vi "TestHarnessDPL-SCPI.vi"() -> ()   [LabVIEW 2025]
uses:
  Program Files/National Instruments/LabVIEW 2024/vi.lib/SmarAct/SmarActCTL/SA_CTL.lvclass
  <vilib>/Utility/miscctls.llb/LVMajorAndMinorColorsTypeDef.ctl
  <vilib>/Analysis/1siggen.llb/Ramp Pattern by Samples.vi
  <vilib>/Analysis/1siggen.llb/Ramp Pattern by Delta.vi
  <vilib>/Analysis/NI_AALBase.lvlib
  <userlib>/_OpenG.lib/time/time.llb/openg_time.lvlib
  instr.lib/Detector SCPI/Detector SCPI.lvlib
  <vilib>/Analysis/NI_AALPro.lvlib
  <vilib>/platform/TimedLoop/XDataNode/XDataNode.xnode
  <vilib>/Platform/TimedLoop/XDataNode/nitl_modes.ctl
  <vilib>/Platform/TimedLoop/XDataNode/XDNodeRunTimeDep.lvlib
  <vilib>/Platform/TimedLoop/XDataNode/wakeup.ctl
  <vilib>/Platform/TimedLoop/XDataNode/timing_clust.ctl
  instr.lib/Keithley 24XX/Keithley 24XX.lvlib
panel:
  out "Ref":dbl[](array[numeric])
  out "SweepData":dbl[][](array[numeric])
  in  "Exit":bool
  out "PositionerStatus":T1={"Moving"=FALSE, "CL Active"=FALSE, "Calibrating"=FALSE, "Referencing"=FALSE, "Delayed Move"=FALSE, "Sensor Present"=TRUE, "Is Calibrated"=TRUE, "Is Referenced"=TRUE, "End Stop"=FALSE, "Ranger Limit"=FALSE, "Following Limit"=FALSE, "Movement Fail"=FALSE, "Is Streaming"=FALSE, "Overload"=FALSE, "Over Temp"=FALSE, "Reference Mark"=FALSE, "Is Phased"=FALSE, "Positioner Fault"=FALSE, "Amplifier Enabled"=TRUE, "In Position"=FALSE, "Brake Enabled"=FALSE}
  out "ChannelState":i32=262368 format="%x"
  in  "Measurement Mode":T2(tab)=enum."Stage Calibration"
  in  "Device Locator":string(combo)="network:sn:MCS2-00005242"
  in  "findDevices":bool caption="Find Devices"
  in  "connect":bool
  out "connected":bool=TRUE
  out "Error Out":errorcluster
  in  "calibrate":bool
  in  "reference":bool
  in  "moveValue":i64=-10400000000 caption="Move Abs (µm)"
  in  "moveMode":u16(ring) caption="Move Mode" items=["CL_ABS", "CL_REL", "SCAN_ABS", "SCAN_REL", "STEP"]
  in  "move":bool
  in  "actuatorMode":enum32{"0", "1"}(radio)
  out "MCSChannel":i8
  out "Position (µm)":dbl=-7999576013.0
  in  "MoveStage":bool
  in  "Move To (mm)":dbl min=-13.5 max=13.5
  in  "Enable":bool=TRUE
  in  "Positioner\n Delay (ms)":u16(ring)=2 items=["1", "2", "5", "10", "20", "50", "100", "200", "500"]
  in  "Delay(mS)":u32=5
  out "Elapsed (ms)":dbl=6.0
  out "Waveform Chart":dbl(graph)=-7999.576013
  out "Peak-to-Peak (µm)":dbl=0.0026870000001508743 format="%^.4g"
  out "rms (µm)":dbl=-2.7284841053187847e-12 format="%^.4g"
  in  "Recalibrate":bool
  out "Calibration":cluster{"Array":dbl[], "Array":dbl[]}(graph)
  in  "Stage\nCal":dbl[][](array[numeric])=[[1020.0, -8440.0], [1100.0, -6120.0], [1200.0, -3330.0], [1300.0, -530.0], [1400.0, 2280.0], [1500.0, 5160.0], [1600.0, 8630.0]]
  out "slope":dbl
  out "intercept":dbl
  in  "SPI Clock":i64
  in  "Oversample":i32=1000 min=1 max=4096
  in  "Power":bool=TRUE
  in  "Detector VISA":refnum<visa-resource-name>="COM4"
  out "Detector Resource":refnum<visa-resource-name>="COM4"
  out "Voltage (V)":dbl[](array[numeric])=[3.264, 0.0, 12.488, 12.77]
  out "Current (mA)":dbl[](array[numeric])=[0.0, 0.0, 21.6, -3.65]
  in  "ThrowAway":i32=100 min=1 max=10000
  out "Detector EGSE ID String":string="Aberystwyth University,Enfys Detector,#01,v0.5.0\r\n"
  in  "ResetVDACstats":bool
  out "Counts":dbl(graph)=160.194
  in  "Gain":u16(ring) items=["High", "Med", "Low"]
  in  "DAC Value":i32=2076 min=0 max=4095 step=1
  in  "Detector":u16(ring) items=["SWIR", "MWIR"]
  out "Peak-to-Peak (counts)":dbl=0.0026870000001508743 format="%^.4g"
  out "rms (counts) 2":dbl=-2.7284841053187847e-12 format="%^.4g"
  out "Mean Value (counts)":dbl
  out "Elapsed(uS)":i32
  in  "Pause":bool
  out "XY Graph":cluster{i32[], "subarray":dbl[]}(graph)
  in  "Detector 3":u16(ring) items=["SWIR", "MWIR"]
  in  "Gain 3":u16(ring) items=["High", "Med", "Low"]
  in  "Grid":bool
  in  "SetSample":bool
  in  "SetRef":bool
  in  "Dark Level":dbl
  out "End(nm)":dbl
  out "Start(nm)":dbl
  out "Sweep":cluster{"Ramp Pattern":dbl[], dbl[]}(graph)
  in  "Go":bool
  in  "Step(µm)":dbl=10.0 min=1.0 max=2000.0 step=1.0
  in  "Finish (mm)":dbl=-8.0 min=-12.0 max=12.0 step=1.0
  in  "Start (mm)":dbl=-12.0 min=-12.0 max=12.0 step=1.0
  in  "milliseconds\n to wait":u32 max=1000
  in  "Detector 2":u16(ring) items=["SWIR", "MWIR"]
  in  "Gain 2":u16(ring) items=["High", "Med", "Low"]
  out "Elapsed(s)":dbl=32.049
  out "Cursor\nlambda":dbl
  out "samples":i32
  out "Step(nm)":dbl
  out "Reference":cluster{"Ramp Pattern":dbl[], dbl[]}(graph)
  out "Reflectance":cluster{"Ramp Pattern":dbl[], dbl[]}(graph)
  in  "Abort":bool
  out "Output vs current":cluster{dbl[], dbl[]}[](graph)
  in  "ISweep":bool
  in  "NPoints":i32=10 min=10 max=10000 step=1
  in  "MaxCurrent":dbl=1e-11 min=1e-11 max=1e-06
  in  "MinCurrent":dbl=1e-12 min=1e-12 max=1e-06
  in  "CurrentSource":refnum<visa-resource-name>="B2901_SourceMeter"
  in  "Detector 4":u16(ring) items=["SWIR", "MWIR"]
  in  "SweepVDAC":bool
  in  "ISource":dbl min=-1e-06 max=1e-06
  in  "VDAC Step":i32=1 min=1 max=100
  in  "VDAC Max":i32 min=0 max=4095
  in  "VDAC Min":i32 min=0 max=4000
  in  "Detector 5":u16(ring) items=["SWIR", "MWIR"]
  out "VDAC Sweep":cluster{dbl[], dbl[]}[](graph)
  in  "Abort SweepVDAC":bool
  in  "Step":bool
  in  "Delay 1 (ms)":i32
  in  "Current 2":dbl
  in  "Current 1":dbl
  in  "Detector 6":u16(ring) items=["SWIR", "MWIR"]
  out "Step Response":cluster{dbl[], "subarray":dbl[]}(graph)
  in  "chan (0)":i32
  in  "stop":bool
  out "Handle":refnum<class "SA_CTL.lvclass">
  out "exit":bool=TRUE
  # "Stage \n(µm)"
  # "Wavelength\n (nm)"
  # "3.3V supply"
  # "Heater"
  # "+12V Supply"
  # "-12V Supply"
  # "Pause button will halt collection and display.\nThis allows graph to be printed etc."
  # "Burst mode is intended to examine behaviour of the ADC\n\nA burst of readings is recorded on the EGSE and then gathered here."
  # "Set current to Current#1. Waits for Delay 1 to stabilise, then switches to current 2 and reads 1000 readings as fast as possible"
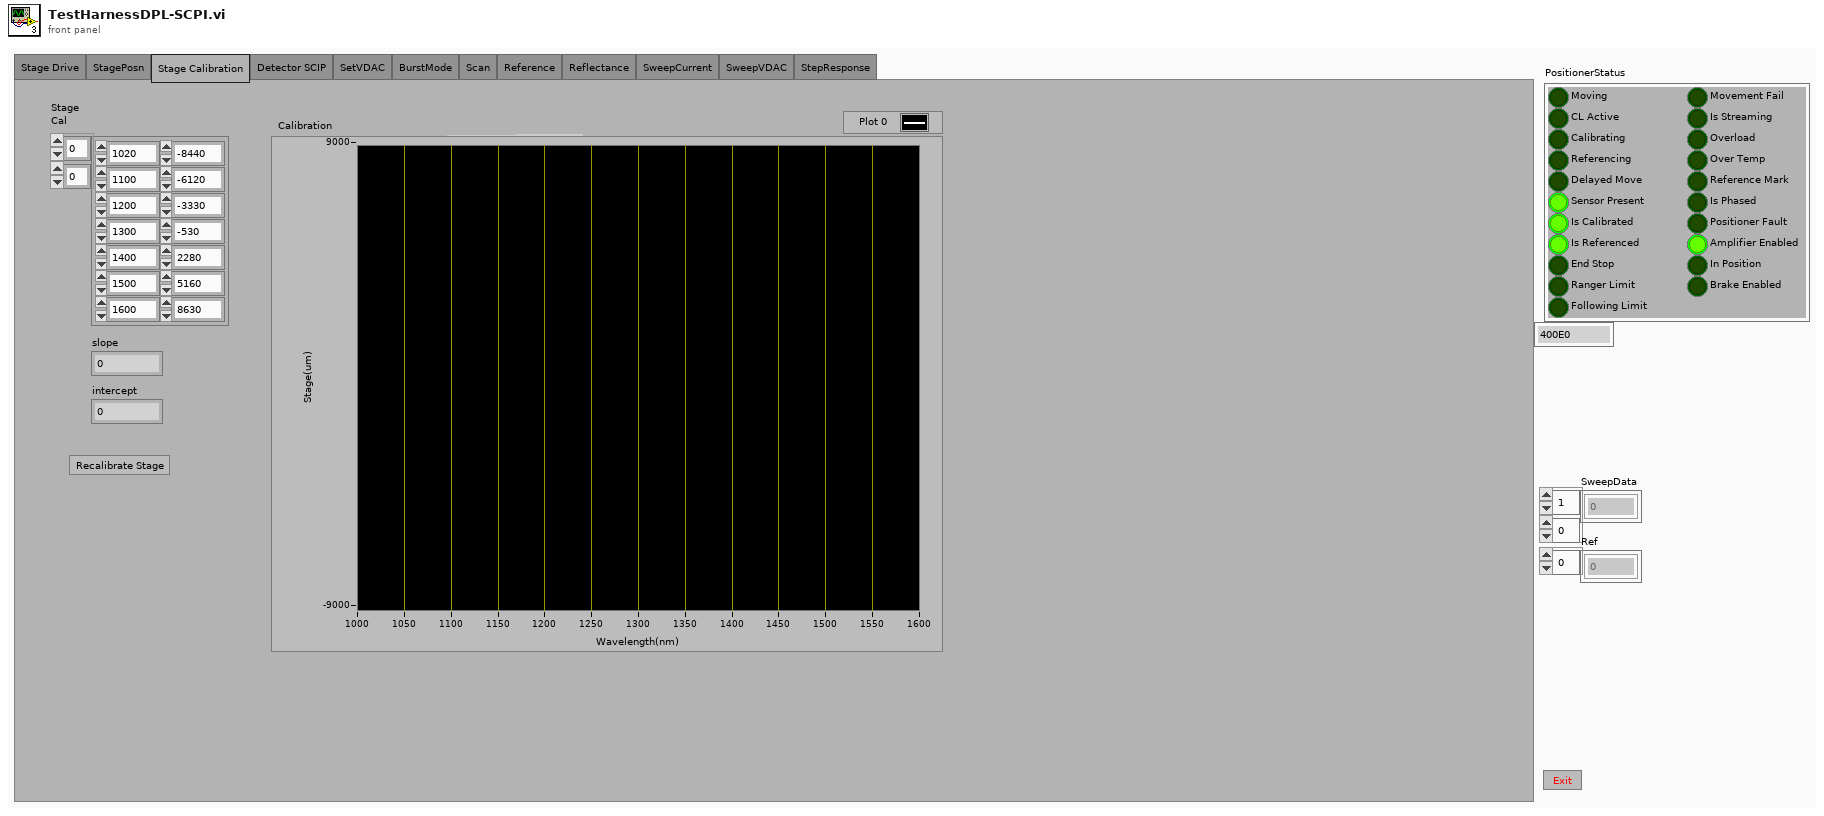
[diagram p1: front panel]
types:
  T1 = cluster{"Moving":bool, "CL Active":bool, "Calibrating":bool, "Referencing":bool, "Delayed Move":bool, "Sensor Present":bool, "Is Calibrated":bool, "Is Referenced":bool, "End Stop":bool, "Ranger Limit":bool, "Following Limit":bool, "Movement Fail":bool, "Is Streaming":bool, "Overload":bool, "Over Temp":bool, "Reference Mark":bool, "Is Phased":bool, "Positioner Fault":bool, "Amplifier Enabled":bool, "In Position":bool, "Brake Enabled":bool}
  T2 = enum32{"Stage Drive", "StagePosn", "Stage Calibration", "Detector SCIP", "SetVDAC", "BurstMode", "Scan", "Reference", "Reflectance", "SweepCurrent", "SweepVDAC", "StepResponse"}
  T3 = enum32{"Stage Drive", "StagePosn", "Stage Calibration", "Detector SCIP", "SetVDAC", "BurstMode", "Scan", "Reference", "Reflectance"}
  T4 = typedef "XDNodeRunTimeDep.lvlib/timing_clust.ctl" = cluster{"Expected End [f-1]":u64, "Actual End [f-1]":u64, "Finished Late? [f-1]":bool, "Expected End [i-1]":u64, "Actual End [i-1]":u64, "Finished Late? [i-1]":bool, "Expected Start [i]":u64, "Actual Start [i]":u64, "Expected Start [f]":u64, "Actual Start [f]":u64, "Source Name":string, "Structure Name":string, "Period":i64, "Deadline":i64, "Offset":i64, "Start":i64, "Priority":i32, "Timeout":i32, "Mode":T5, "Wakeup Reason":T6, "Error":errorcluster, "Source Type":string, "Secondary Source Type":string, "Global End Time":u64, "Global Start Time":u64, "Frame Duration":u64, "Iteration Duration":u64, "Assigned CPU":i32, "I/O Scan Engine Mode":u32}
  T5 = typedef "XDNodeRunTimeDep.lvlib/nitl_modes.ctl" = enum32{"No Change", "Process missed periods, maintain original phase", "Discard missed periods, maintain original phase", "Process missed periods, ignore original phase", "Discard missed periods, ignore original phase"}
  T6 = typedef "XDNodeRunTimeDep.lvlib/wakeup.ctl" = enum32{"Normal", "Aborted", "Asynchronous wakeup", "Timing source error", "Timed loop error", "Timeout"}
  T7 = typedef "LVMajorAndMinorColorsTypeDef.ctl" = cluster{"Major Color":u32, "Minor Color":u32}
  T8 = cluster{"Boolean array[0]":bool, "Boolean array[1]":bool, "Boolean array[2]":bool, "Boolean array[3]":bool, "Boolean array[4]":bool, "Boolean array[5]":bool, "Boolean array[6]":bool, "Boolean array[7]":bool, "Boolean array[8]":bool, "Boolean array[9]":bool, "Boolean array[10]":bool, "Boolean array[11]":bool, "Boolean array[12]":bool, "Boolean array[13]":bool, "Boolean array[14]":bool, "Boolean array[15]":bool, "Boolean array[16]":bool, "Boolean array[17]":bool, "Boolean array[18]":bool, "Boolean array[19]":bool, "Boolean array[20]":bool}
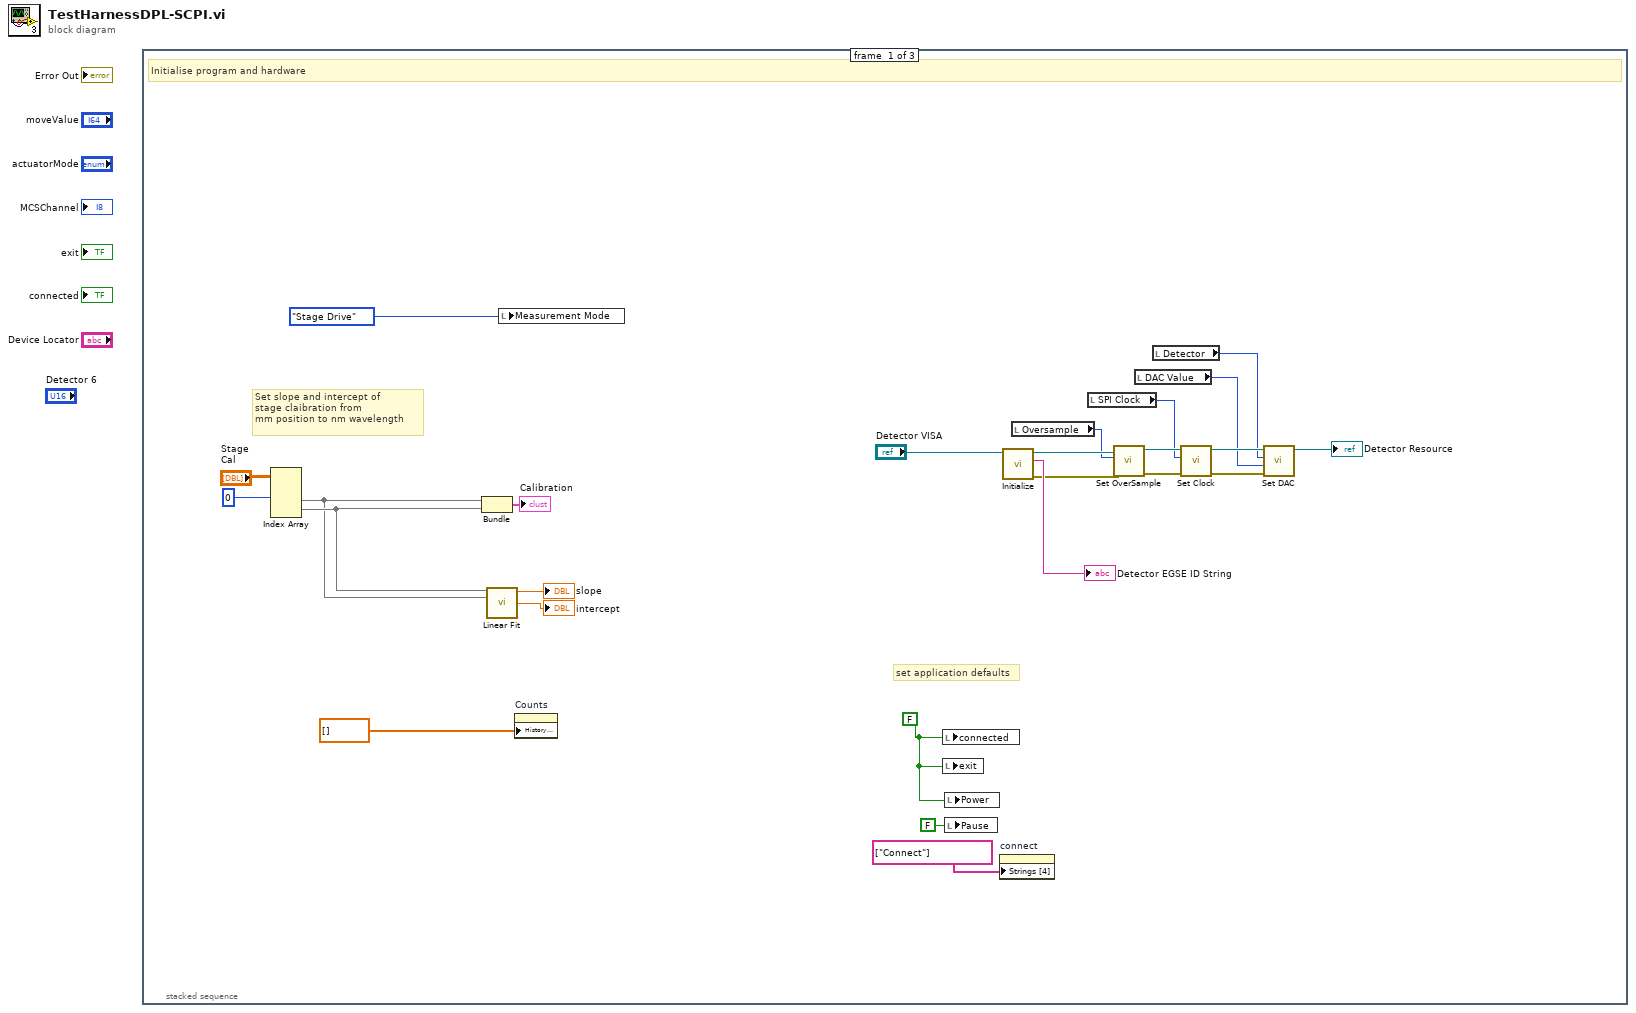
[diagram p0: block diagram]
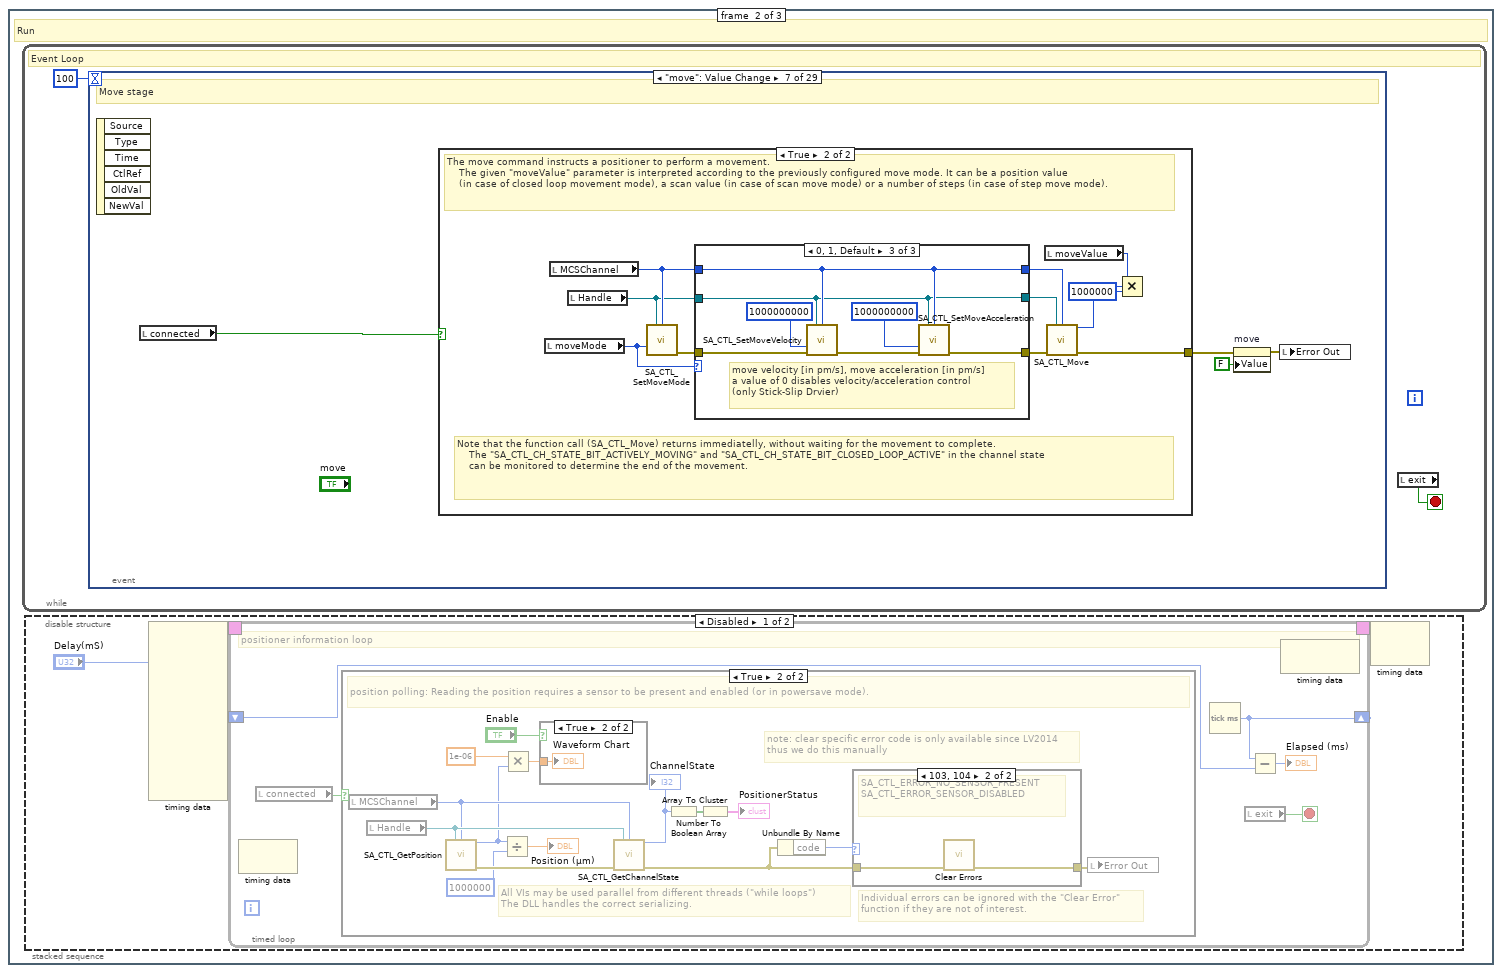
[diagram p2: hidden frame]
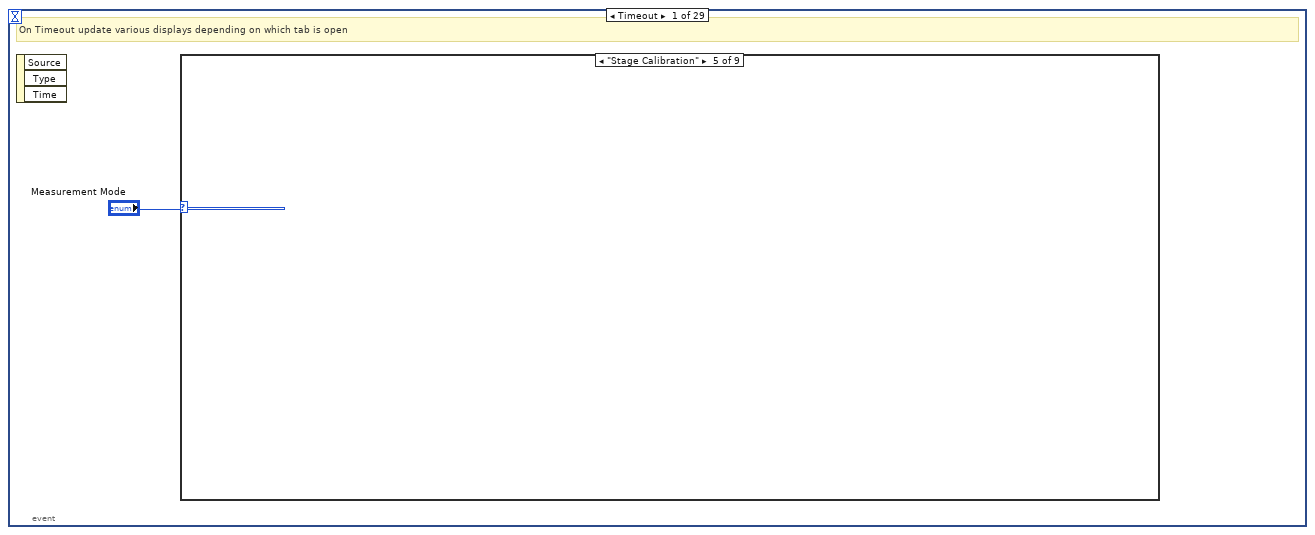
[diagram p7: hidden frame]
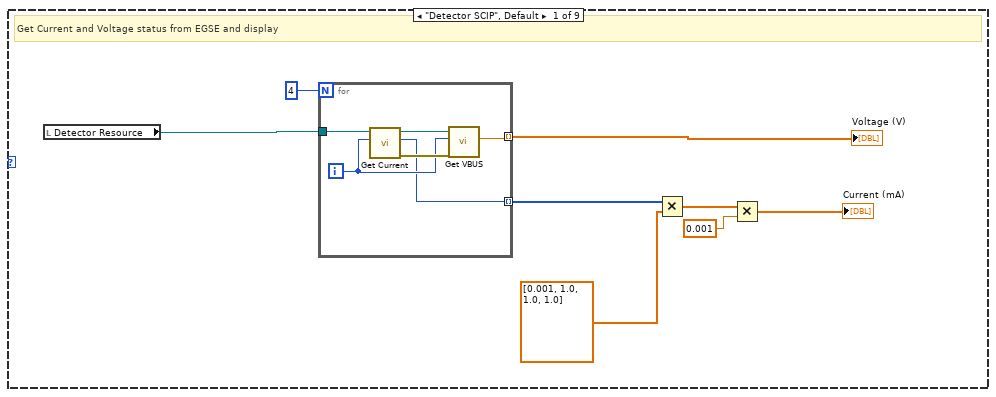
[diagram p8: hidden frame]
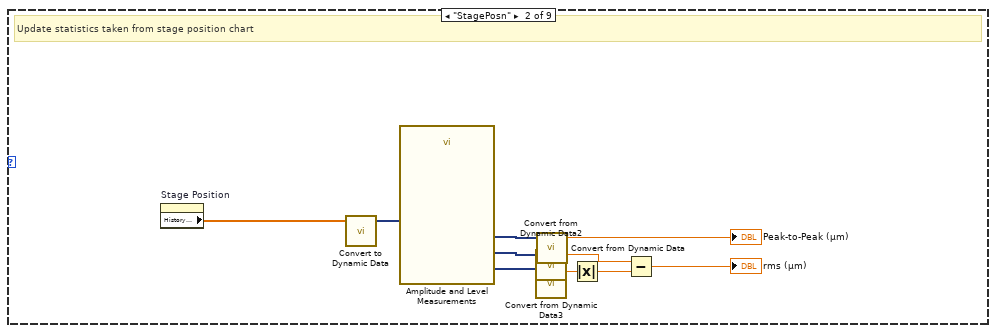
[diagram p9: hidden frame]
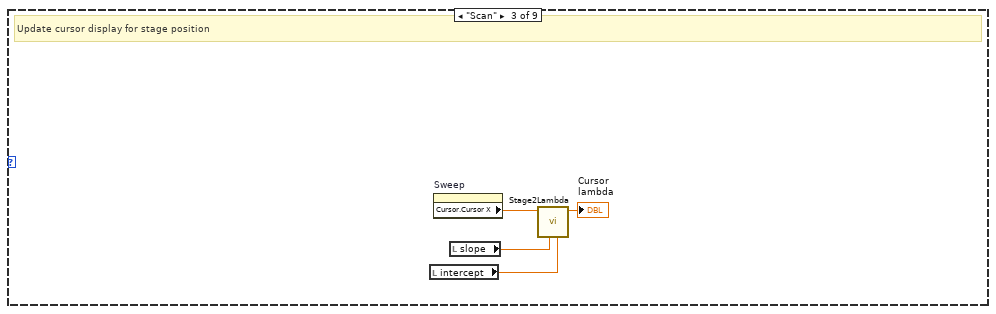
[diagram p10: hidden frame]
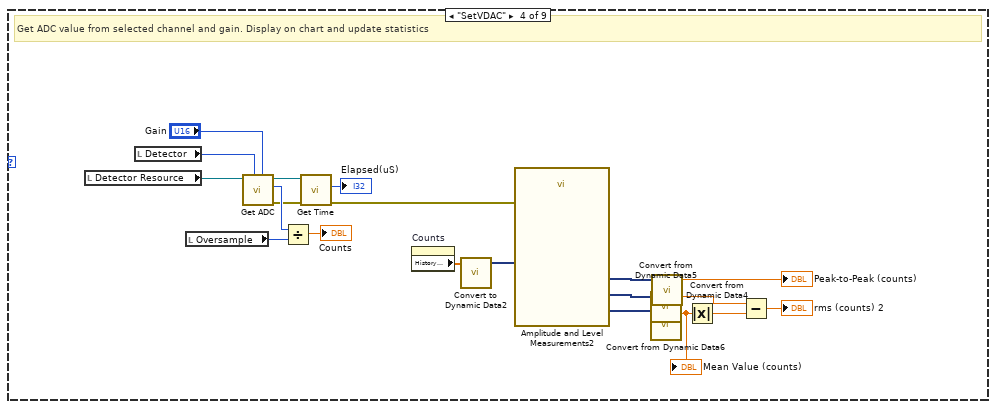
[diagram p11: hidden frame]
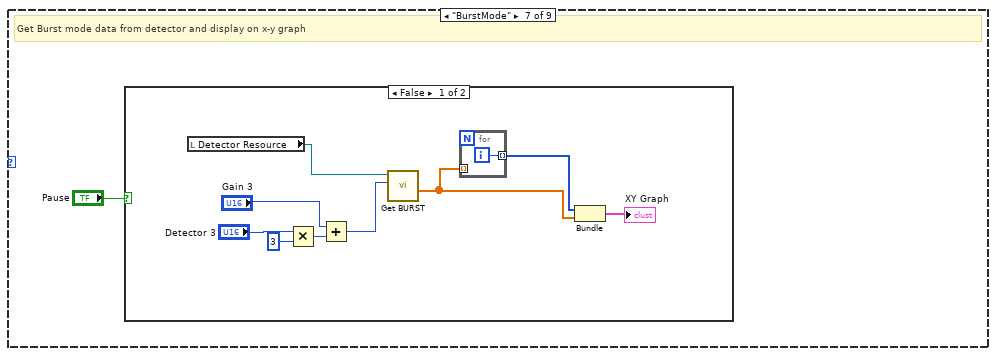
[diagram p13: hidden frame]
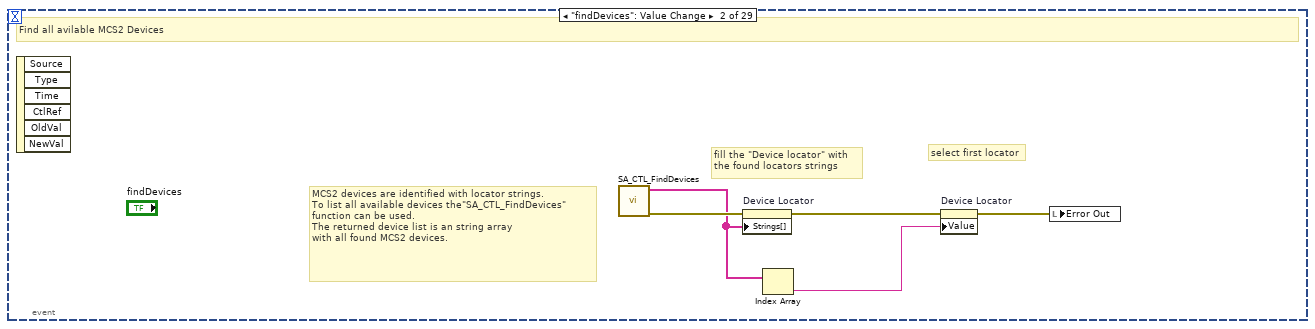
[diagram p17: hidden frame]
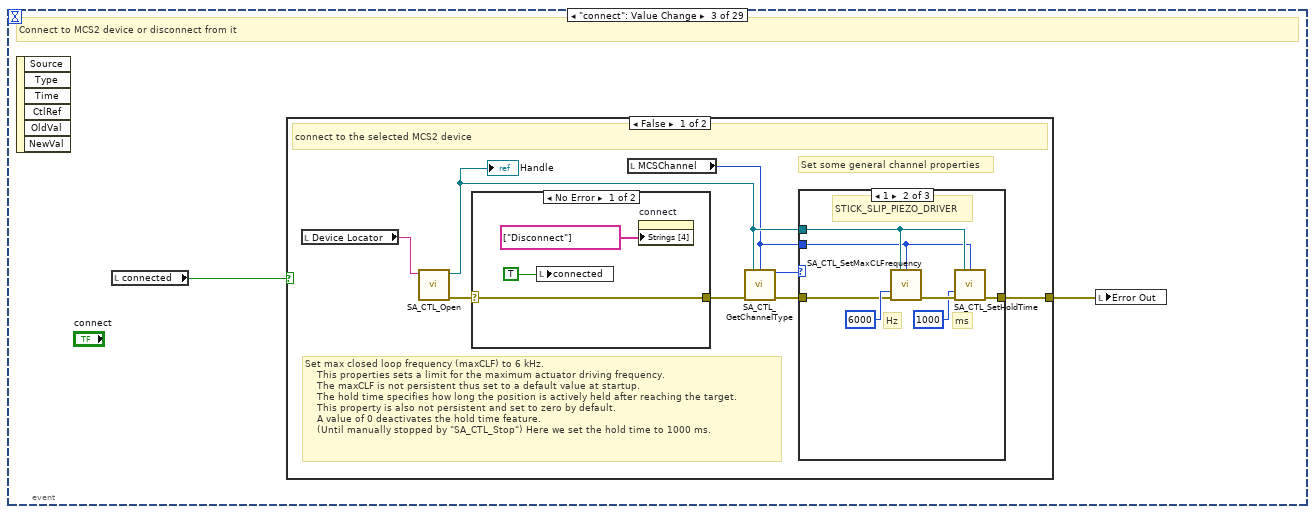
[diagram p18: hidden frame]
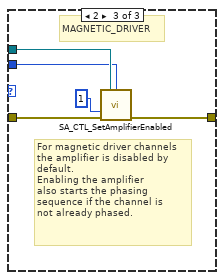
[diagram p20: hidden frame]
diagram:
  n1 = stacked-sequence {
    frame #0 {
      w21 = FALSE ("connected")
      # "Set slope and intercept of \nstage claibration from\nmm position to nm wavelength"
      # "set application defaults"
      # "Initialise program and hardware"
      n2 = Index Array(array="Stage\nCal", index (col) #1=0 ("disabled index (col)")) -> (element #1=w17:dbl[], element #2=w18:dbl[])  [unwired: 3 in]
      n3 = Bundle("Stage\nCal"=w17, "Stage\nCal"=w18) -> (→"Calibration":cluster{"Stage\nCal":dbl[], "Stage\nCal":dbl[]})  [unwired: 1 in]
      n4 = call <vilib>:"Linear Fit.vi"("Y"=w18, "X"=w17) -> ("slope"=→"slope":dbl, "intercept"=→"intercept":dbl)  [unwired: 9 in, 3 out]
      n5 = local write "Measurement Mode"(T3."Stage Drive" ("Tab Control")) -> ()
      n6 = property on="Counts" class="WFChart (strict)"("History Data"=dbl[] []) -> ()  [unwired: 2 in, 2 out]
      n7 = local write "connected"(w21) -> ()
      n8 = local write "exit"(w21) -> ()
      n9 = local write "Power"(w21) -> ()
      n10 = local write "Pause"(FALSE ("Pause")) -> ()
      n11 = property on="connect" class="Bool"("Strings [4]"=string[] ["Connect"]) -> ()  [unwired: 2 in, 2 out]
      n12 = call "Initialize.vi"("VISA resource name"="Detector VISA") -> ("error out"=w10:errorcluster, "ID String"=→"Detector EGSE ID String":string, "VISA resource name out"=w9:refnum<visa-resource-name>)  [unwired: 8 in]
      n13 = local read "Oversample"() -> (w8:i32)
      n14 = local read "SPI Clock"() -> (w3:i64)
      n15 = call "Set OverSample.vi"("error in (no error)"=w10, "oversample (0)"=w8, "VISA resource name"=w9) -> ("error out"=w7:errorcluster, "VISA resource name out"=w5:refnum<visa-resource-name>)  [unwired: 7 in]
      n16 = local read "DAC Value"() -> (w1:i32)
      n17 = local read "Detector"() -> (w2:u16)
      n18 = call "Set Clock.vi"("error in (no error)"=w7, "ClockSpeed"=w3, "VISA resource name"=w5) -> ("error out"=w6:errorcluster, "VISA resource name out"=w4:refnum<visa-resource-name>)  [unwired: 7 in]
      n19 = call "Set DAC.vi"("error in (no error)"=w6, "value (0)"=w1, "chan (0)"=w2, "VISA resource name"=w4) -> ("VISA resource name out"=→"Detector Resource":refnum<visa-resource-name>)  [unwired: 6 in, 1 out]
    }
    frame #1 {
      # "Run"
      n20 = while {
        stop <- w59 stop-if-true
        # "Event Loop"
        n21 = event shown="[6] \"move\": Value Change" {
          selector: _ -> [_ _ _ _ _ _ _ _ _ _ _ _ _ _ _ _ _ _ _ _ _ _ _ _ _ _ _ _ _]
          dyn-events: _ -> [_ _ _ _ _ _ _ _ _ _ _ _ _ _ _ _ _ _ _ _ _ _ _ _ _ _ _ _ _]
          timeout: 100 -> [_ _ _ _ _ _ _ _ _ _ _ _ _ _ _ _ _ _ _ _ _ _ _ _ _ _ _ _ _]
          event Timeout {
            # "On Timeout update various displays depending on which tab is open"
            n22 = event-data() -> ()  [unwired: 1 in, 3 out]
            n23 = case shown="\"Stage Calibration\"" "Measurement Mode" {
              frame "Detector SCIP", Default {
                # "Get Current and Voltage status from EGSE and display"
                n24 = local read "Detector Resource"() -> (w69:refnum<visa-resource-name>)
                n25 = for {
                  N: 4 -> [_]
                  tunnel: w69 -> [w75]
                  tunnel: [w71] -> w66 mode=indexing
                  tunnel: [w70] -> w67 mode=indexing
                  i -> [w72]
                  n26 = call "Get Current.vi"("chan (1)"=w72, "VISA resource name"=w75) -> ("error out"=w74:errorcluster, "output"=w71:i32, "VISA resource name out"=w73:refnum<visa-resource-name>)  [unwired: 7 in]
                  n27 = call "Get VBUS.vi"("error in (no error)"=w74, "chan (1)"=w72, "VISA resource name"=w73) -> ("output"=w70:dbl)  [unwired: 6 in, 2 out]
                }
                "Voltage (V)" <- w67
                n28 = Multiply(x=w66, y=dbl[] [0.001, 1.0, 1.0, 1.0]) -> (x*y=w63:dbl[])
                n29 = Multiply(x=w63, y=0.001) -> (x*y=→"Current (mA)":dbl[])
              }
              frame "StagePosn" {
                # "Update statistics taken from stage position chart"
                n30 = property on="Stage Position" class="WFChart (strict)"() -> ("History Data"=w85:dbl[])  [unwired: 2 in, 2 out]
                n31 = call "Convert to Dynamic Data"("Array"=w85) -> ("Dynamic Data Type"=w84:dynamicdata)  [unwired: 3 in]
                n32 = call "Amplitude and Level Measurements"("Signals"=w84) -> ("Mean (DC)"=w79:dynamicdata, "RMS"=w80:dynamicdata, "Peak to Peak"=w83:dynamicdata)  [unwired: 11 in, 1 out]
                n33 = call "Convert from Dynamic Data2"("Dynamic Data Type"=w80) -> ("Scalar"=w81:dbl)  [unwired: 3 in]
                n34 = call "Convert from Dynamic Data3"("Dynamic Data Type"=w79) -> ("Scalar"=w78:dbl)  [unwired: 3 in]
                n35 = call "Convert from Dynamic Data"("Dynamic Data Type"=w83) -> ("Scalar"=→"Peak-to-Peak (µm)":dbl)  [unwired: 3 in]
                n36 = Absolute Value(x=w78) -> (abs(x)=w76:dbl)
                n37 = Subtract(x=w81, y=w76) -> (x-y=→"rms (µm)":dbl)
              }
              frame "Scan" {
                # "Update cursor display for stage position"
                n38 = local read "intercept"() -> (w87:dbl)
                n39 = property on="Sweep" class="XYGraph (strict)"() -> ("Cursor.Cursor X"=w89:dbl)  [unwired: 2 in, 2 out]
                n40 = local read "slope"() -> (w88:dbl)
                n41 = call "Stage2Lambda.vi"("intercept"=w87, "slope"=w88, "Stage (mm)"=w89) -> ("lambda"=→"Cursor\nlambda":dbl)  [unwired: 8 in]
              }
              frame "SetVDAC" {
                # "Get ADC value from selected channel and gain. Display on chart and update statistics"
                n42 = local read "Detector Resource"() -> (w109:refnum<visa-resource-name>)
                n43 = local read "Detector"() -> (w104:u16)
                n44 = local read "Oversample"() -> (w106:i32)
                n45 = call "Get ADC.vi"("Gain"="Gain", "Detector"=w104, "VISA resource name"=w109) -> ("error out"=w102:errorcluster, "output"=w108:i32, "VISA resource name out"=w103:refnum<visa-resource-name>)  [unwired: 6 in]
                n46 = Divide(x=w108, y=w106) -> (x/y=→"Counts":dbl)
                n47 = call "Get Time.vi"("error in (no error)"=w102, "VISA resource name"=w103) -> ("error out"=w90:errorcluster, "output"=→"Elapsed(uS)":i32)  [unwired: 7 in, 1 out]
                n48 = property on="Counts" class="WFChart (strict)"() -> ("History Data"=w100:dbl[])  [unwired: 2 in, 2 out]
                n49 = call "Convert to Dynamic Data2"("Array"=w100) -> ("Dynamic Data Type"=w91:dynamicdata)  [unwired: 3 in]
                n50 = call "Amplitude and Level Measurements2"("Signals"=w91, "error in (no error)"=w90) -> ("Mean (DC)"=w96:dynamicdata, "RMS"=w95:dynamicdata, "Peak to Peak"=w92:dynamicdata)  [unwired: 10 in, 1 out]
                n51 = call "Convert from Dynamic Data5"("Dynamic Data Type"=w95) -> ("Scalar"=w94:dbl)  [unwired: 3 in]
                n52 = call "Convert from Dynamic Data6"("Dynamic Data Type"=w96) -> ("Scalar"=w97:dbl)  [unwired: 3 in]
                "Mean Value (counts)" <- w97
                n53 = call "Convert from Dynamic Data4"("Dynamic Data Type"=w92) -> ("Scalar"=→"Peak-to-Peak (counts)":dbl)  [unwired: 3 in]
                n54 = Absolute Value(x=w97) -> (abs(x)=w99:dbl)
                n55 = Subtract(x=w94, y=w99) -> (x-y=→"rms (counts) 2":dbl)
              }
              frame "Stage Calibration" {
              }
              frame "Stage Drive" {
              }
              frame "BurstMode" {
                # "Get Burst mode data from detector and display on x-y graph"
                n56 = case shown="False" "Pause" {
                  frame False {
                    n57 = local read "Detector Resource"() -> (w119:refnum<visa-resource-name>)
                    n58 = Multiply(x="Detector 3", y=u16 3) -> (x*y=w118:u16)
                    n59 = Add(x="Gain 3", y=w118) -> (x+y=w116:u16)
                    n60 = call "Get BURST.vi"("chan (0)"=w116, "VISA resource name"=w119) -> ("subarray"=w111:dbl[])  [unwired: 6 in, 3 out]
                    n61 = for {
                      tunnel: w111 -> [_] mode=indexing
                      tunnel: [w120] -> w112 mode=indexing
                      i -> [w120]
                    }
                    n62 = Bundle(w112, "subarray"=w111) -> (→"XY Graph":cluster{i32[], "subarray":dbl[]})  [unwired: 1 in]
                  }
                  frame True {
                  }
                }
              }
              frame "Reference" {
              }
              frame "Reflectance" {
              }
            }
          }
          event "findDevices": Value Change {
            # "select first locator"
            # "fill the \"Device locator\" with\nthe found locators strings"
            # "MCS2 devices are identified with locator strings.\nTo list all available devices the\"SA_CTL_FindDevices\"\nfunction can be used.\nThe returned device list is an string array \nwith all found MCS2 devices."
            # "Find all avilable MCS2 Devices"
            n63 = event-data() -> ()  [unwired: 1 in, 6 out]
            n64 = call "SA_CTL_FindDevices.vi"() -> ("error out"=w125:errorcluster, "devices"=w124:string[])  [unwired: 10 in]
            n65 = property on="Device Locator" class="CmbBox"(error in=w125, "Strings[]"=w124) -> (error out=w123:errorcluster)  [unwired: 1 in, 1 out]
            n66 = Index Array(array=w124) -> (element=w122:string)  [unwired: 1 in]
            n67 = property on="Device Locator" class="CmbBox"(error in=w123, "Value"=w122) -> (error out=w121:errorcluster)  [unwired: 1 in, 1 out]
            n68 = local write "Error Out"(w121) -> ()
          }
          event "connect": Value Change {
            # "Connect to MCS2 device or disconnect from it"
            n69 = event-data() -> ()  [unwired: 1 in, 6 out]
            n70 = local read "connected"() -> (w127:bool)
            n71 = case shown="False" w127 {
              tunnel: [w133 w153] -> w126
              frame False {
                # "Set max closed loop frequency (maxCLF) to 6 kHz.\n    This properties sets a limit for the maximum actuator driving frequency.\n    The maxCLF is not persistent thus set to a default value at startup.\n    The hold time specifies how long the position is actively held after reaching the target.\n    This property is also not persistent and set to zero by default.\n    A value of 0 deactivates the hold time feature.\n    (Until manually stopped by \"SA_CTL_Stop\") Here we set the hold time to 1000 ms."
                # "Set some general channel properties"
                # "connect to the selected MCS2 device"
                n72 = local read "Device Locator"() -> (w134:string)
                n73 = call "SA_CTL_Open.vi"("locator"=w134) -> ("error out"=w135:errorcluster, "SA_CTL_Handle"=w129:refnum<class "SA_CTL.lvclass">)  [unwired: 9 in]
                "Handle" <- w129
                n74 = case shown="No Error" w135 {
                  selector: w135 -> [w149 w152]
                  tunnel: [w149 w152] -> w132
                  frame No Error {
                    n75 = local write "connected"(TRUE ("connected")) -> ()
                    n76 = property on="connect" class="Bool"("Strings [4]"=string[] ["Disconnect"]) -> ()  [unwired: 2 in, 2 out]
                  }
                  frame Error {
                  }
                }
                n77 = local read "MCSChannel"() -> (w128:i8)
                n78 = call "SA_CTL_GetChannelType.vi"("SA_CTL_Handle"=w129, "channel"=w128, "error in (no error)"=w132) -> ("ChannelType"=w131:i32, "error out"=w130:errorcluster)  [unwired: 11 in]
                n79 = case shown="1" w131 {
                  tunnel: w129 -> [_ w140 w145]
                  tunnel: [w136 w139 w147] -> w133
                  tunnel: w128 -> [_ w138 w144]
                  tunnel: w130 -> [w136 w137 w148]
                  frame 0, Default {
                    # "unknown"
                  }
                  frame 1 {
                    # "Hz"
                    # "ms"
                    # "STICK_SLIP_PIEZO_DRIVER"
                    n80 = call "SA_CTL_SetMaxCLFrequency.vi"("SA_CTL_Handle"=w140, "channel"=w138, "MaxCLFrequency"=6000 ("MaxCLF"), "error in (no error)"=w137) -> ("error out"=w143:errorcluster)  [unwired: 11 in]
                    n81 = call "SA_CTL_SetHoldTime.vi"("SA_CTL_Handle"=w140, "channel"=w138, "HoldTime"=1000 ("MaxCLF"), "error in (no error)"=w143) -> ("error out"=w139:errorcluster)  [unwired: 11 in]
                  }
                  frame 2 {
                    # "For magnetic driver channels\nthe amplifier is disabled by\ndefault. \nEnabling the amplifier\nalso starts the phasing\nsequence if the channel is\nnot already phased."
                    # "MAGNETIC_DRIVER"
                    n82 = call "SA_CTL_SetAmplifierEnabled.vi"("SA_CTL_Handle"=w145, "channel"=w144, "AmplifierEnabled"=1, "error in (no error)"=w148) -> ("error out"=w147:errorcluster)  [unwired: 11 in]
                  }
                }
              }
              frame True {
                # "disconnect the MCS2 device"
                n83 = local read "Handle"() -> (w156:refnum<class "SA_CTL.lvclass">)
                n84 = call "SA_CTL_Close.vi"("SA_CTL_Handle"=w156) -> ("error out"=w153:errorcluster)  [unwired: 10 in]
                n85 = local write "connected"(FALSE ("connected")) -> ()
                n86 = property on="connect" class="Bool"("Strings [4]"=string[] ["Connect"]) -> ()  [unwired: 2 in, 2 out]
              }
            }
            n87 = local write "Error Out"(w126) -> ()
          }
          event "stop": Value Change {
            # "Stop - stop any movement on MCS2"
            n88 = event-data() -> ()  [unwired: 1 in, 6 out]
            n89 = local read "connected"() -> (w158:bool)
            n90 = case shown="True" w158 {
              tunnel: [_ w161] -> w157
              frame False {
              }
              frame True {
                # "Note for closed loop movements with acceleration control enabled:\n\n    The first \"stop\" command sent while moving triggers the positioner to come to a halt by decellerating to zero.\n    A second \"stop\" command triggers a hard stop (\"emergency stop\")."
                # "This command stops any ongoing movement. It also stops the hold position feature of a closed loop command."
                n91 = local read "MCSChannel"() -> (w159:i8)
                n92 = local read "Handle"() -> (w160:refnum<class "SA_CTL.lvclass">)
                n93 = call "SA_CTL_Stop.vi"("SA_CTL_Handle"=w160, "channel"=w159) -> ("error out"=w161:errorcluster)  [unwired: 13 in]
              }
            }
            n94 = local write "Error Out"(w157) -> ()
          }
          event "calibrate": Value Change {
            # "Calibratre MCS2"
            n95 = event-data() -> ()  [unwired: 1 in, 6 out]
            n96 = local read "connected"() -> (w163:bool)
            n97 = case shown="True" w163 {
              tunnel: [_ w168] -> w162
              frame False {
              }
              frame True {
                # "calibration options:\nstartDirection forward"
                # "Note that the function call (SA_CTL_Calibrate) returns immediatelly, without waiting for the movement to complete.\n    The \"SA_CTL_CH_STATE_BIT_CALIBRATING\" in the channel state can be monitored to determine the end of the calibration\n    sequence. \n \n WARNING\n    During the calibration sequence the positioner performs a movement of up to several mm, make sure to not start\n    the calibration near a mechanical endstop in order to ensure proper operation."
                # "The calibration sequence is used to increase the precision of the position calculation. This function should be called once for each\n    channel if the mechanical setup changes. (e.g. a different positioner was connected to the channel, the positioner type was set to a \n    different type) The calibration data will be saved to non-volatile memory, thus it is not necessaray to perform the calibration sequence\n    on each initialization. Note: the \"SA_CTL_CH_STATE_BIT_IS_CALIBRATED\" in the channel state can be used to determine\n    if valid calibration data is stored for the specific channel."
                n98 = local read "MCSChannel"() -> (w165:i8)
                n99 = local read "Handle"() -> (w166:refnum<class "SA_CTL.lvclass">)
                n100 = call "SA_CTL_SetCalibrationOptions.vi"("SA_CTL_Handle"=w166, "channel"=w165, "CalibrationOptions"=0 ("CalibrationMode")) -> ("error out"=w167:errorcluster)  [unwired: 12 in]
                n101 = call "SA_CTL_Calibrate.vi"("handle"=w166, "channel"=w165, "error in (no error)"=w167) -> ("error out"=w168:errorcluster)  [unwired: 12 in]
              }
            }
            n102 = local write "Error Out"(w162) -> ()
          }
          event "reference": Value Change {
            # "Find reference mark on stage"
            n103 = event-data() -> ()  [unwired: 1 in, 6 out]
            n104 = local read "connected"() -> (w170:bool)
            n105 = case shown="True" w170 {
              tunnel: [_ w179] -> w169
              frame False {
              }
              frame True {
                # "Note for Stick-Slip Driver:\nSetting the acceleration to zero \ndisables the acceleration control."
                # "The reference options specifies the behaviour of the find reference sequence. The reference flags can be ORed to build the \n    reference options. By default (options = 0) the positioner returns to the position of the reference mark.\n    Note: In contrast to previous controller systems this is not mandatory. The MCS2 controller is able to find the reference\n    position \"on-the-fly\". See the MCS2 Programmer Guide for a description of the different modes.\n    Note that the  function call (SA_CTL_Reference) returns immediatelly, without waiting for the movement to complete.\n    The \"SA_CTL_CH_STATE_BIT_REFERENCING\" in the channel state can be monitored to determine the end of the referencing\n    sequence.\n    Gere we use the \"autoZero\" option to set the position to zero after the reference position was found."
                # "Since the position sensors work on an incremental base, the referencing sequence is used to establish an absolute positioner \n    reference for the positioner after system startup.\n    Note: the \"SA_CTL_CH_STATE_BIT_IS_REFERENCED\" in the channel state can be used to to decide whether it is necessary\n    to perform the referencing sequence."
                n106 = local read "MCSChannel"() -> (w174:i8)
                n107 = local read "Handle"() -> (w175:refnum<class "SA_CTL.lvclass">)
                n108 = call "SA_CTL_SetReferencingOptions.vi"("SA_CTL_Handle"=w175, "channel"=w174, "ReferencingOptions"=0 ("CalibrationMode")) -> ("error out"=w177:errorcluster)  [unwired: 12 in]
                n109 = call "SA_CTL_SetMoveVelocity.vi"("SA_CTL_Handle"=w175, "channel"=w174, "MoveVelocity"=i64 1000000000 ("FindReferenceVelocity"), "error in (no error)"=w177) -> ("error out"=w178:errorcluster)  [unwired: 11 in]
                n110 = call "SA_CTL_SetMoveAcceleration.vi"("SA_CTL_Handle"=w175, "channel"=w174, "MoveAcceleration"=i64 10000000000 ("FindReferenceAcceleration"), "error in (no error)"=w178) -> ("error out"=w176:errorcluster)  [unwired: 11 in]
                n111 = call "SA_CTL_Reference.vi"("SA_CTL_Handle"=w175, "channel"=w174, "error in (no error)"=w176) -> ("error out"=w179:errorcluster)  [unwired: 12 in]
              }
            }
            n112 = local write "Error Out"(w169) -> ()
          }
          event "move": Value Change {
            # "Move stage"
            n113 = event-data() -> ()  [unwired: 1 in, 6 out]
            n114 = local read "connected"() -> (w183:bool)
            n115 = case shown="True" w183 {
              tunnel: [_ w194] -> w182
              frame False {
              }
              frame True {
                # "Note that the function call (SA_CTL_Move) returns immediatelly, without waiting for the movement to complete.\n    The \"SA_CTL_CH_STATE_BIT_ACTIVELY_MOVING\" and \"SA_CTL_CH_STATE_BIT_CLOSED_LOOP_ACTIVE\" in the channel state \n    can be monitored to determine the end of the movement."
                # "The move command instructs a positioner to perform a movement.\n    The given \"moveValue\" parameter is interpreted according to the previously configured move mode. It can be a position value\n    (in case of closed loop movement mode), a scan value (in case of scan move mode) or a number of steps (in case of step move mode)."
                n116 = local read "moveMode"() -> (w188:u16)
                n117 = local read "MCSChannel"() -> (w191:i8)
                n118 = local read "Handle"() -> (w186:refnum<class "SA_CTL.lvclass">)
                n119 = call "SA_CTL_SetMoveMode.vi"("SA_CTL_Handle"=w186, "channel"=w191, "MoveMode"=w188) -> ("error out"=w193:errorcluster)  [unwired: 12 in]
                n120 = case shown="0, 1, Default" w188 {
                  tunnel: w193 -> [w199 w205 w212]
                  tunnel: [w196 w202 w211] -> w192
                  tunnel: w191 -> [w198 w204 w208]
                  tunnel: [w198 w204 w208] -> w190
                  tunnel: w186 -> [w197 w203 w207]
                  tunnel: [w197 w203 w207] -> w189
                  frame 2, 3 {
                    # "scan velocity [in dac increments/s]"
                    n121 = call "SA_CTL_SetScanVelocity.vi"("SA_CTL_Handle"=w197, "channel"=w198, "ScanVelocity"=i64 65535, "error in (no error)"=w199) -> ("error out"=w196:errorcluster)  [unwired: 11 in]
                  }
                  frame 4 {
                    # "step amplitude [in dac incr.]\n0 to 65535 -> 0 to 100 V"
                    # "step frequency [in Hz]\nvalid range: 1 to 20000 Hz"
                    n122 = call "SA_CTL_SetStepFrequency.vi"("SA_CTL_Handle"=w203, "channel"=w204, "StepFrequency"=1000, "error in (no error)"=w205) -> ("error out"=w206:errorcluster)  [unwired: 11 in]
                    n123 = call "SA_CTL_SetStepAmplitude.vi"("SA_CTL_Handle"=w203, "channel"=w204, "StepAmplitude"=65535, "error in (no error)"=w206) -> ("error out"=w202:errorcluster)  [unwired: 11 in]
                  }
                  frame 0, 1, Default {
                    # "move velocity [in pm/s], move acceleration [in pm/s]\na value of 0 disables velocity/acceleration control\n(only Stick-Slip Drvier)"
                    n124 = call "SA_CTL_SetMoveVelocity.vi"("SA_CTL_Handle"=w207, "channel"=w208, "MoveVelocity"=i64 1000000000 ("FindReferenceVelocity"), "error in (no error)"=w212) -> ("error out"=w213:errorcluster)  [unwired: 11 in]
                    n125 = call "SA_CTL_SetMoveAcceleration.vi"("SA_CTL_Handle"=w207, "channel"=w208, "MoveAcceleration"=i64 1000000000 ("FindReferenceVelocity"), "error in (no error)"=w213) -> ("error out"=w211:errorcluster)  [unwired: 11 in]
                  }
                }
                n126 = local read "moveValue"() -> (w187:i64)
                n127 = Multiply(x=w187, y=i64 1000000) -> (x*y=w185:i64)
                n128 = call "SA_CTL_Move.vi"("moveValue"=w185, "SA_CTL_Handle"=w189, "channel"=w190, "error in (no error)"=w192) -> ("error out"=w194:errorcluster)  [unwired: 11 in]
              }
            }
            n129 = property on="move" class="Bool (strict)"(error in=w182, "Value"=FALSE ("move")) -> (error out=w181:errorcluster)  [unwired: 1 in, 1 out]
            n130 = local write "Error Out"(w181) -> ()
          }
          event "moveMode": Value Change {
            # "Put correct text in caption of MoveValue control"
            n131 = event-data() -> ()  [unwired: 1 in, 6 out]
            n132 = Index Array(array=string[] ["Move Abs (pm)", "Move Rel (pm)", "Move Value", "Move Value", "Move (steps)"], index="moveMode") -> (element=w215:string)
            n133 = property on="moveValue" class="DigNum (strict)"("Caption.Text"=w215) -> ()  [unwired: 2 in, 2 out]
          }
          event "actuatorMode": Value Change {
            # "Set Actuator Mode - Quiet/Normal"
            n134 = event-data() -> ("NewVal"=w217:enum32{"0", "1"})  [unwired: 1 in, 5 out]
            n135 = local read "connected"() -> (w219:bool)
            n136 = case shown="True" w219 {
              tunnel: [_ w222] -> w218
              tunnel: w217 -> [_ w220]
              frame False {
              }
              frame True {
                # "The actuator mode specifies the type of driving signal generation.\n        - normal mode (0) :    the control loop generates actuator driving signals with a maximum frequency limited to the max closed loop \n                                               frequency (maxCLF).\n        - quiet mode (1):        allows positioner movement with minimal noise emission.\n    Note that this property is not available for Magnetic Driver channels."
                n137 = local read "MCSChannel"() -> (w223:i8)
                n138 = local read "Handle"() -> (w221:refnum<class "SA_CTL.lvclass">)
                n139 = call "SA_CTL_SetActuatorMode.vi"("SA_CTL_Handle"=w221, "channel"=w223, "ActuatorMode"=w220) -> ("error out"=w222:errorcluster)  [unwired: 12 in]
              }
            }
            n140 = local write "Error Out"(w218) -> ()
          }
          event "Positioner\n Delay (ms)": Value Change {
            # "Sets delay between reading stage positioner"
            n141 = event-data() -> ()  [unwired: 1 in, 6 out]
            n142 = property on="Positioner\n Delay (ms)" class="Ring (strict)"() -> ("Strings []"=w227:string[])  [unwired: 2 in, 2 out]
            n143 = Index Array(array=w227, index="Positioner\n Delay (ms)") -> (element=w226:string)
            n144 = Decimal String To Number(string=w226) -> (number=w225:i32)  [unwired: 2 in, 1 out]
            n145 = local write "Delay(mS)"(w225) -> ()
          }
          event "Power": Value Change {
            # "Use SCPI to turn power to detector board on/off"
            n146 = event-data() -> ()  [unwired: 1 in, 6 out]
            n147 = local read "Detector Resource"() -> (w229:refnum<visa-resource-name>)
            n148 = call "Set Power.vi"("Power (0)"="Power", "VISA resource name"=w229) -> ()  [unwired: 8 in, 2 out]
          }
          event "SPI Clock": Value Change {
            n149 = event-data() -> ()  [unwired: 1 in, 6 out]
            n150 = local read "Detector Resource"() -> (w231:refnum<visa-resource-name>)
            n151 = call "Set Clock.vi"("ClockSpeed"="SPI Clock", "VISA resource name"=w231) -> ()  [unwired: 8 in, 2 out]
          }
          event "ResetVDACstats": Value Change {
            # "Reset statistics on SetVDAC page"
            n152 = event-data() -> ()  [unwired: 1 in, 6 out]
            n153 = property on="Counts" class="WFChart (strict)"("History Data"=dbl[] []) -> ()  [unwired: 2 in, 2 out]
          }
          event "Recalibrate": Value Change {
            # "Update slope and intercept for stageposn<=>lambda calculations from \"Stage Cal\" control"
            n154 = event-data() -> ()  [unwired: 1 in, 6 out]
            n155 = local read "Stage\nCal"() -> (w237:dbl[][])
            n156 = Index Array(array=w237, index (col) #1=0 ("disabled index (col)")) -> (element #1=w238:dbl[], element #2=w239:dbl[])  [unwired: 3 in]
            n157 = Bundle("Stage\nCal"=w238, "Stage\nCal"=w239) -> (w235:cluster{"Stage\nCal":dbl[], "Stage\nCal":dbl[]})  [unwired: 1 in]
            n158 = call <vilib>:"Linear Fit.vi"("Y"=w239, "X"=w238) -> ("slope"=w234:dbl, "intercept"=w233:dbl)  [unwired: 9 in, 3 out]
            n159 = local write "Calibration"(w235) -> ()
            n160 = local write "slope"(w234) -> ()
            n161 = local write "intercept"(w233) -> ()
          }
          event "MoveStage": Value Change {
            # "1E9 converts mm to pm"
            # "Move stage in mm"
            n162 = event-data() -> ()  [unwired: 1 in, 6 out]
            n163 = local read "MCSChannel"() -> (w244:i8)
            n164 = local read "Handle"() -> (w240:refnum<class "SA_CTL.lvclass">)
            n165 = Multiply(x="Move To (mm)", y=1000000000.0) -> (x*y=w242:dbl)
            n166 = To Quad Integer(1:w242) -> (0:w241:i64)
            n167 = call "SA_CTL_Move.vi"("moveValue"=w241, "SA_CTL_Handle"=w240, "channel"=w244) -> ()  [unwired: 12 in, 1 out]
          }
          event "Oversample": Value Change {
            # "Change Oversample value on EGSE"
            n168 = event-data() -> ()  [unwired: 1 in, 6 out]
            n169 = local read "Detector Resource"() -> (w247:refnum<visa-resource-name>)
            n170 = call "Set OverSample.vi"("oversample (0)"="Oversample", "VISA resource name"=w247) -> ()  [unwired: 8 in, 2 out]
          }
          event "ThrowAway": Value Change {
            # "Change Throwaway value on EGSE"
            n171 = event-data() -> ()  [unwired: 1 in, 6 out]
            n172 = local read "Detector Resource"() -> (w249:refnum<visa-resource-name>)
            n173 = call "Set ThrowAway.vi"("ThrowAway (0)"="ThrowAway", "VISA resource name"=w249) -> ()  [unwired: 8 in, 2 out]
          }
          event "DAC Value": Value Change {
            # "Change offset DAC on selected channel of detector card"
            n174 = event-data() -> ()  [unwired: 1 in, 6 out]
            n175 = local read "Detector Resource"() -> (w250:refnum<visa-resource-name>)
            n176 = call "Set DAC.vi"("value (0)"="DAC Value", "chan (0)"="Detector", "VISA resource name"=w250) -> ()  [unwired: 7 in, 2 out]
          }
          event "Go": Value Change {
            # "Initiate stage sweep"
            n177 = event-data() -> ()  [unwired: 1 in, 6 out]
            n178 = case shown="True" "Go" {
              frame False {
              }
              frame True {
                n179 = property on="Sweep" class="XYGraph (strict)"("ActXScl"=0 ("Active X Scale")) -> (error out=w258:errorcluster)  [unwired: 2 in, 1 out]
                n180 = local read "MCSChannel"() -> (w270:i8)
                n181 = local read "Handle"() -> (w269:refnum<class "SA_CTL.lvclass">)
                n182 = call <userlib>:"Tick Count (ms)__ogtk.vi"("error in (no error)"=w258) -> ("error out"=w266:errorcluster, "millisecond timer value"=w263:u32)  [unwired: 9 in]
                n183 = call "SA_CTL_SetMoveVelocity.vi"("SA_CTL_Handle"=w269, "channel"=w270, "MoveVelocity"=i64 0, "error in (no error)"=w266) -> ("error out"=w274:errorcluster)  [unwired: 11 in]
                n184 = Multiply(x=0.001, y="Step(µm)") -> (x*y=w276:dbl)
                n185 = call-poly <vilib>:"Ramp Pattern.vi"("start"="Start (mm)", "end"="Finish (mm)", "delta"=w276) -> ("samples"=→"samples":i32, "Ramp Pattern"=w267:dbl[])  [unwired: 6 in, 1 out]
                n186 = call "SA_CTL_SetMoveAcceleration.vi"("SA_CTL_Handle"=w269, "channel"=w270, "MoveAcceleration"=i64 0 ("FindReferenceVelocity"), "error in (no error)"=w274) -> ("error out"=w272:errorcluster)  [unwired: 11 in]
                n187 = for {
                  tunnel: w267 -> [w314] mode=indexing
                  tunnel: w270 -> [w310]
                  tunnel: w269 -> [w309]
                  tunnel: w272 -> [w306]
                  shift-right: [w303] -> w256
                  shift-left: dbl[] [] -> [w305]
                  tunnel: w267 -> [w296]
                  tunnel: [w297] -> w265
                  tunnel: [w296] -> w257
                  n188 = property on="Sweep" class="XYGraph (strict)"() -> (error out=w295:errorcluster, "ActXScl"=w293:i32)  [unwired: 2 in, 1 out]
                  n189 = Multiply(x=1000000000.0, y=w314) -> (x*y=w312:dbl)
                  n190 = call "SA_CTL_Move.vi"("moveValue"=w312, "SA_CTL_Handle"=w309, "channel"=w310, "error in (no error)"=w306) -> ("error out"=w311:errorcluster)  [unwired: 11 in]
                  n191 = property on="Sweep" class="XYGraph (strict)"(error in=w295, "ActXScl"=0 ("Active X Scale")) -> (error out=w294:errorcluster)  [unwired: 1 in, 1 out]
                  n192 = while {
                    tunnel: w311 -> [w322]
                    tunnel: w310 -> [w321]
                    tunnel: w309 -> [w320]
                    tunnel: [w316] -> w308
                    stop <- w318 stop-if-true
                    n193 = call "SA_CTL_GetChannelState.vi"("SA_CTL_Handle"=w320, "channel"=w321, "error in (no error)"=w322) -> ("ChannelState"=w319:i32, "error out"=w316:errorcluster)  [unwired: 11 in]
                    n194 = And(x=1, y=w319) -> (x .and. y?=w315:i32)
                    n195 = Equal To 0?(x=w315) -> (x = 0?=w318:bool)
                  }
                  n196 = property on="Sweep" class="XYGraph (strict)"(error in=w294) -> (error out=w292:errorcluster, "XScale.Maximum"=w289:dbl, "XScale.Minimum"=w287:dbl)  [unwired: 1 in, 1 out]
                  n197 = local read "intercept"() -> (w285:dbl)
                  n198 = local read "slope"() -> (w284:dbl)
                  n199 = call <userlib>:"Wait (ms)__ogtk.vi"("error in (no error)"=w308, "milliseconds to wait"="milliseconds\n to wait") -> ("error out"=w298:errorcluster)  [unwired: 8 in, 1 out]
                  n200 = property on="Sweep" class="XYGraph (strict)"(error in=w292, "ActXScl"=1 ("Active X Scale")) -> (error out=w290:errorcluster)  [unwired: 1 in, 1 out]
                  n201 = local read "Detector Resource"() -> (w299:refnum<visa-resource-name>)
                  n202 = local read "Oversample"() -> (w300:i32)
                  n203 = call "Stage2Lambda.vi"("intercept"=w285, "slope"=w284, "Stage (mm)"=w289) -> ("lambda"=w288:dbl)  [unwired: 8 in]
                  n204 = call "Stage2Lambda.vi"("intercept"=w285, "slope"=w284, "Stage (mm)"=w287) -> ("lambda"=w286:dbl)  [unwired: 8 in]
                  n205 = call "Get ADC.vi"("Gain"="Gain 2", "Detector"="Detector 2", "error in (no error)"=w298, "VISA resource name"=w299) -> ("error out"=w297:errorcluster, "output"=w302:i32)  [unwired: 5 in, 1 out]
                  n206 = property on="Sweep" class="XYGraph (strict)"(error in=w290, "XScale.Maximum"=w288, "XScale.Minimum"=w286) -> (error out=w291:errorcluster)  [unwired: 1 in, 1 out]
                  n207 = Divide(x=w302, y=w300) -> (x/y=w301:dbl)
                  n208 = Build Array (concatenate)(w305, w301) -> (w303:dbl[])
                  n209 = Bundle("Ramp Pattern"=w296, w303) -> (→"Sweep":cluster{"Ramp Pattern":dbl[], dbl[]})  [unwired: 1 in]
                  n210 = property on="Sweep" class="XYGraph (strict)"(error in=w291, "ActXScl"=w293) -> ()  [unwired: 1 in, 2 out]
                }
                n211 = call <userlib>:"Tick Count (ms)__ogtk.vi"("error in (no error)"=w265) -> ("millisecond timer value"=w264:u32)  [unwired: 9 in, 1 out]
                n212 = Build Array(w257, w256) -> (→"SweepData":dbl[][])
                n213 = Subtract(x=w264, y=w263) -> (x-y=w262:u32)
                n214 = Multiply(x=0.001, y=w262) -> (x*y=→"Elapsed(s)":dbl)
              }
            }
          }
          event "Start (mm)", "Finish (mm)": Value Change {
            n215 = event-data() -> ()  [unwired: 1 in, 6 out]
            n216 = local read "slope"() -> (w327:dbl)
            n217 = local read "Start (mm)"() -> (w328:dbl)
            n218 = local read "intercept"() -> (w326:dbl)
            n219 = call "Stage2Lambda.vi"("intercept"=w326, "slope"=w327, "Stage (mm)"=w328) -> ("lambda"=→"Start(nm)":dbl)  [unwired: 8 in]
            n220 = local read "Finish (mm)"() -> (w325:dbl)
            n221 = call "Stage2Lambda.vi"("intercept"=w326, "slope"=w327, "Stage (mm)"=w325) -> ("lambda"=→"End(nm)":dbl)  [unwired: 8 in]
          }
          event "Grid": Value Change {
            # "Turn graph grid on/off"
            n222 = event-data() -> ()  [unwired: 1 in, 6 out]
            n223 = case shown="True" "Grid" {
              tunnel: [1 0] -> w333
              tunnel: [0 1] -> w332
              frame True {
              }
              frame False {
              }
            }
            n224 = property on="Sweep" class="XYGraph (strict)"() -> (error out=w331:errorcluster, "ActXScl"=w329:i32)  [unwired: 2 in, 1 out]
            n225 = property on="Sweep" class="XYGraph (strict)"(error in=w331, "ActXScl"=w333) -> (error out=w339:errorcluster)  [unwired: 1 in, 1 out]
            n226 = property on="Sweep" class="XYGraph (strict)"(error in=w339, "XScale.GridColors"=T7 {"Major Color"=0, "Minor Color"=0} ("X Scale.Grid Colors")) -> (error out=w337:errorcluster)  [unwired: 1 in, 1 out]
            n227 = property on="Sweep" class="XYGraph (strict)"(error in=w337, "ActXScl"=w332) -> (error out=w336:errorcluster)  [unwired: 1 in, 1 out]
            n228 = property on="Sweep" class="XYGraph (strict)"(error in=w336, "XScale.GridColors"=T7 {"Major Color"=10066176, "Minor Color"=5000192} ("X Scale.Grid Colors")) -> (error out=w330:errorcluster)  [unwired: 1 in, 1 out]
            n229 = property on="Sweep" class="XYGraph (strict)"(error in=w330, "ActXScl"=w329) -> ()  [unwired: 1 in, 2 out]
          }
          event "Step(µm)": Value Change {
            n230 = event-data() -> ("NewVal"=w346:dbl)  [unwired: 1 in, 5 out]
            n231 = local read "slope"() -> (w345:dbl)
            n232 = Divide(x=w346, y=w345) -> (x/y=→"Step(nm)":dbl)
          }
          event "SetRef": Value Change {
            # "Set Reference Spectrum"
            n233 = event-data() -> ()  [unwired: 1 in, 6 out]
            n234 = case shown="True" "SetRef" {
              frame False {
              }
              frame True {
                n235 = local read "SweepData"() -> (w354:dbl[][])
                n236 = Index Array(array=w354, index (row) #1=0 ("disabled index (col)")) -> (element #1=w351:dbl[], element #2=w353:dbl[])  [unwired: 3 in]
                n237 = Subtract(x=w353, y="Dark Level") -> (x-y=w350:dbl[])
                "Ref" <- w350
                n238 = Bundle("SweepData"=w351, w350) -> (→"Reference":cluster{"SweepData":dbl[], dbl[]})  [unwired: 1 in]
              }
            }
          }
          event "SetSample": Value Change {
            # "Copy current spectrum as Sample"
            n239 = event-data() -> ()  [unwired: 1 in, 6 out]
            n240 = case shown="True" "SetSample" {
              frame False {
              }
              frame True {
                n241 = local read "SweepData"() -> (w365:dbl[][])
                n242 = local read "Dark Level"() -> (w363:dbl)
                n243 = Index Array(array=w365, index (row) #1=0 ("disabled index (col)")) -> (element #1=w360:dbl[], element #2=w364:dbl[])  [unwired: 3 in]
                n244 = local read "Ref"() -> (w361:dbl[])
                n245 = Subtract(x=w364, y=w363) -> (x-y=w362:dbl[])
                n246 = Divide(x=w362, y=w361) -> (x/y=w358:dbl[])
                n247 = for {
                  tunnel: w360 -> [w369] mode=indexing
                  tunnel: [w366] -> w359 mode=indexing
                  n248 = local read "intercept"() -> (w367:dbl)
                  n249 = local read "slope"() -> (w368:dbl)
                  n250 = call "Stage2Lambda.vi"("intercept"=w367, "slope"=w368, "Stage (mm)"=w369) -> ("lambda"=w366:dbl)  [unwired: 8 in]
                }
                n251 = Bundle(w359, w358) -> (→"Reflectance":cluster{dbl[], dbl[]})  [unwired: 1 in]
              }
            }
          }
          event "ISweep": Value Change {
            n252 = event-data() -> ()  [unwired: 1 in, 6 out]
            n253 = case shown="True" "ISweep" {
              frame False {
              }
              frame True {
                w378 = u16 1 items=["Voltage", "Current"] ("Source Mode  (0: Voltage)")
                w383 = dbl[] []
                w400 = u16 1 items=["Voltage", "Current"] ("Source Mode  (0: Voltage)")
                w404 = u16 1 items=["Volts", "Current", "Resistance"] ("Function (0: Volts)")
                w406 = u16 0 items=["Volts", "Current", "Resistance"] ("Function (0: Volts)")
                n254 = call "Initialize.vi"("ID Query (True)"=FALSE, "VISA resource name"="CurrentSource") -> ("error out"=w391:errorcluster, "VISA resource name out"=w392:refnum<visa-resource-name>)  [unwired: 8 in]
                n255 = Logarithm Base 10(1:"MaxCurrent") -> (0:w382:dbl)
                n256 = Logarithm Base 10(1:"MinCurrent") -> (0:w381:dbl)
                n257 = call "Configure Measurement.vi"("error in (no error)"=w391, "Enable Auto Range (T:Enable)"=TRUE, "Function (0: Volts)"=w406, "VISA resource name"=w392) -> ("error out"=w407:errorcluster, "VISA resource name out"=w408:refnum<visa-resource-name>)  [unwired: 6 in]
                n258 = call "Configure Measurement.vi"("Manual Range (1.0)"=1e-07, "error in (no error)"=w407, "Enable Auto Range (T:Enable)"=FALSE, "Function (0: Volts)"=w404, "VISA resource name"=w408) -> ("error out"=w402:errorcluster, "VISA resource name out"=w401:refnum<visa-resource-name>)  [unwired: 5 in]
                n259 = call-poly <vilib>:"Ramp Pattern.vi"("start"=w381, "end"=w382, "samples"="NPoints") -> ("Ramp Pattern"=w385:dbl[])  [unwired: 7 in, 1 out]
                n260 = local read "Oversample"() -> (w379:i32)
                n261 = local read "Detector Resource"() -> (w384:refnum<visa-resource-name>)
                n262 = call "Configure Output.vi"("Source Mode  (0: Voltage)"=w400, "error in (no error)"=w402, "Output Level (0)"=0.0, "VISA resource name"=w401) -> ("error out"=w398:errorcluster, "VISA resource name out"=w397:refnum<visa-resource-name>)  [unwired: 6 in]
                n263 = Power Of 10(x=w385) -> (10^x=w380:dbl[])
                n264 = call "Enable Output.vi"("error in (no error)"=w398, "Enable Output (T: Enable)"=TRUE, "VISA resource name"=w397) -> ("error out"=w394:errorcluster, "VISA resource name out"=w395:refnum<visa-resource-name>)  [unwired: 7 in]
                n265 = for {
                  tunnel: w395 -> [w444]
                  tunnel: w394 -> [w445]
                  tunnel: w380 -> [w443] mode=indexing
                  tunnel: [w441] -> w377
                  tunnel: [w432] -> w375
                  shift-right: [w436] -> _
                  shift-left: w383 -> [w438]
                  tunnel: w380 -> [w423]
                  tunnel: w384 -> [w435]
                  shift-right: [w425] -> _
                  shift-left: w383 -> [w427]
                  shift-right: [w424] -> _
                  shift-left: w383 -> [w426]
                  tunnel: w379 -> [w413]
                  tunnel: "Detector 4" -> [w411]
                  stop <- "Abort" stop-if-true
                  w428 = u16 2 items=["High", "Med", "Low"] ("Gain")
                  w429 = u16 1 items=["High", "Med", "Low"] ("Gain")
                  w439 = u16 0 items=["High", "Med", "Low"] ("Gain")
                  w442 = u16 1 items=["Voltage", "Current"] ("Source Mode  (0: Voltage)")
                  n266 = call "Configure Output.vi"("Source Mode  (0: Voltage)"=w442, "error in (no error)"=w445, "Output Level (0)"=w443, "VISA resource name"=w444) -> ("error out"=w440:errorcluster, "VISA resource name out"=w441:refnum<visa-resource-name>)  [unwired: 6 in]
                  n267 = call "Get ADC.vi"("Gain"=w439, "Detector"=w411, "error in (no error)"=w440, "VISA resource name"=w435) -> ("error out"=w434:errorcluster, "output"=w437:i32, "VISA resource name out"=w431:refnum<visa-resource-name>)  [unwired: 5 in]
                  n268 = Divide(x=w437, y=w413) -> (x/y=w417:dbl)
                  n269 = call "Get ADC.vi"("Gain"=w429, "Detector"=w411, "error in (no error)"=w434, "VISA resource name"=w431) -> ("error out"=w433:errorcluster, "output"=w416:i32, "VISA resource name out"=w430:refnum<visa-resource-name>)  [unwired: 5 in]
                  n270 = Divide(x=w416, y=w413) -> (x/y=w415:dbl)
                  n271 = call "Get ADC.vi"("Gain"=w428, "Detector"=w411, "error in (no error)"=w433, "VISA resource name"=w430) -> ("error out"=w432:errorcluster, "output"=w412:i32)  [unwired: 5 in, 1 out]
                  n272 = Divide(x=w412, y=w413) -> (x/y=w414:dbl)
                  n273 = Build Array (concatenate)(w427, w415) -> (w425:dbl[])
                  n274 = Build Array (concatenate)(w438, w417) -> (w436:dbl[])
                  n275 = Build Array (concatenate)(w426, w414) -> (w424:dbl[])
                  n276 = Bundle(w423, w436) -> (w422:cluster{dbl[], dbl[]})  [unwired: 1 in]
                  n277 = Bundle(w423, w425) -> (w421:cluster{dbl[], dbl[]})  [unwired: 1 in]
                  n278 = Bundle(w423, w424) -> (w420:cluster{dbl[], dbl[]})  [unwired: 1 in]
                  n279 = Build Array(w422, w421, w420) -> (→"Output vs current":cluster{dbl[], dbl[]}[])
                }
                n280 = call "Configure Output.vi"("Source Mode  (0: Voltage)"=w378, "error in (no error)"=w375, "Output Level (0)"=0.0, "VISA resource name"=w377) -> ("error out"=w374:errorcluster, "VISA resource name out"=w376:refnum<visa-resource-name>)  [unwired: 6 in]
                n281 = call "Enable Output.vi"("error in (no error)"=w374, "Enable Output (T: Enable)"=FALSE, "VISA resource name"=w376) -> ("error out"=w390:errorcluster, "VISA resource name out"=w389:refnum<visa-resource-name>)  [unwired: 7 in]
                n282 = call "Close.vi"("error in (no error)"=w390, "VISA resource name"=w389) -> ()  [unwired: 9 in, 1 out]
              }
            }
          }
          event "SweepVDAC": Value Change {
            n283 = event-data() -> ()  [unwired: 1 in, 6 out]
            n284 = case shown="True" "SweepVDAC" {
              frame False {
              }
              frame True {
                w459 = u16 1 items=["Voltage", "Current"] ("Source Mode  (0: Voltage)")
                w461 = dbl[] []
                w474 = u16 1 items=["Voltage", "Current"] ("Source Mode  (0: Voltage)")
                w478 = u16 1 items=["Volts", "Current", "Resistance"] ("Function (0: Volts)")
                w480 = u16 0 items=["Volts", "Current", "Resistance"] ("Function (0: Volts)")
                n285 = local read "CurrentSource"() -> (w452:refnum<visa-resource-name>)
                n286 = call "Initialize.vi"("ID Query (True)"=FALSE, "VISA resource name"=w452) -> ("error out"=w466:errorcluster, "VISA resource name out"=w467:refnum<visa-resource-name>)  [unwired: 8 in]
                n287 = call "Configure Measurement.vi"("error in (no error)"=w466, "Enable Auto Range (T:Enable)"=TRUE, "Function (0: Volts)"=w480, "VISA resource name"=w467) -> ("error out"=w481:errorcluster, "VISA resource name out"=w482:refnum<visa-resource-name>)  [unwired: 6 in]
                n288 = call "Configure Measurement.vi"("Manual Range (1.0)"=1e-07, "error in (no error)"=w481, "Enable Auto Range (T:Enable)"=FALSE, "Function (0: Volts)"=w478, "VISA resource name"=w482) -> ("error out"=w476:errorcluster, "VISA resource name out"=w475:refnum<visa-resource-name>)  [unwired: 5 in]
                n289 = call-poly <vilib>:"Ramp Pattern.vi"("start"="VDAC Min", "end"="VDAC Max", "delta"="VDAC Step") -> ("Ramp Pattern"=w463:dbl[])  [unwired: 6 in, 2 out]
                n290 = local read "Oversample"() -> (w460:i32)
                n291 = local read "Detector Resource"() -> (w462:refnum<visa-resource-name>)
                n292 = call "Configure Output.vi"("Source Mode  (0: Voltage)"=w474, "error in (no error)"=w476, "Output Level (0)"="ISource", "VISA resource name"=w475) -> ("error out"=w473:errorcluster, "VISA resource name out"=w472:refnum<visa-resource-name>)  [unwired: 6 in]
                n293 = call "Enable Output.vi"("error in (no error)"=w473, "Enable Output (T: Enable)"=TRUE, "VISA resource name"=w472) -> ("error out"=w469:errorcluster, "VISA resource name out"=w470:refnum<visa-resource-name>)  [unwired: 7 in]
                n294 = for {
                  tunnel: w470 -> [w486]
                  tunnel: w469 -> [w517]
                  tunnel: w463 -> [w516] mode=indexing
                  tunnel: [w486] -> w458
                  tunnel: [w508] -> w456
                  shift-right: [w511] -> _
                  shift-left: w461 -> [w513]
                  tunnel: w463 -> [w499]
                  tunnel: w462 -> [w485]
                  shift-right: [w501] -> _
                  shift-left: w461 -> [w503]
                  shift-right: [w500] -> _
                  shift-left: w461 -> [w502]
                  tunnel: w460 -> [w489]
                  tunnel: "Detector 5" -> [w487]
                  stop <- "Abort SweepVDAC" stop-if-true
                  w504 = u16 2 items=["High", "Med", "Low"] ("Gain")
                  w505 = u16 1 items=["High", "Med", "Low"] ("Gain")
                  w514 = u16 0 items=["High", "Med", "Low"] ("Gain")
                  n295 = call "Set DAC.vi"("error in (no error)"=w517, "value (0)"=w516, "chan (0)"=w487, "VISA resource name"=w485) -> ("error out"=w515:errorcluster, "VISA resource name out"=w484:refnum<visa-resource-name>)  [unwired: 6 in]
                  n296 = call "Get ADC.vi"("Gain"=w514, "Detector"=w487, "error in (no error)"=w515, "VISA resource name"=w484) -> ("error out"=w510:errorcluster, "output"=w512:i32, "VISA resource name out"=w507:refnum<visa-resource-name>)  [unwired: 5 in]
                  n297 = Divide(x=w512, y=w489) -> (x/y=w493:dbl)
                  n298 = call "Get ADC.vi"("Gain"=w505, "Detector"=w487, "error in (no error)"=w510, "VISA resource name"=w507) -> ("error out"=w509:errorcluster, "output"=w492:i32, "VISA resource name out"=w506:refnum<visa-resource-name>)  [unwired: 5 in]
                  n299 = Divide(x=w492, y=w489) -> (x/y=w491:dbl)
                  n300 = call "Get ADC.vi"("Gain"=w504, "Detector"=w487, "error in (no error)"=w509, "VISA resource name"=w506) -> ("error out"=w508:errorcluster, "output"=w488:i32)  [unwired: 5 in, 1 out]
                  n301 = Divide(x=w488, y=w489) -> (x/y=w490:dbl)
                  n302 = Build Array (concatenate)(w503, w491) -> (w501:dbl[])
                  n303 = Build Array (concatenate)(w513, w493) -> (w511:dbl[])
                  n304 = Build Array (concatenate)(w502, w490) -> (w500:dbl[])
                  n305 = Bundle("Ramp Pattern"=w499, w511) -> (w498:cluster{"Ramp Pattern":dbl[], dbl[]})  [unwired: 1 in]
                  n306 = Bundle("Ramp Pattern"=w499, w501) -> (w497:cluster{"Ramp Pattern":dbl[], dbl[]})  [unwired: 1 in]
                  n307 = Bundle("Ramp Pattern"=w499, w500) -> (w496:cluster{"Ramp Pattern":dbl[], dbl[]})  [unwired: 1 in]
                  n308 = Build Array(w498, w497, w496) -> (→"VDAC Sweep":cluster{"Ramp Pattern":dbl[], dbl[]}[])
                }
                n309 = call "Configure Output.vi"("Source Mode  (0: Voltage)"=w459, "error in (no error)"=w456, "Output Level (0)"=0.0, "VISA resource name"=w458) -> ("error out"=w455:errorcluster, "VISA resource name out"=w457:refnum<visa-resource-name>)  [unwired: 6 in]
                n310 = call "Enable Output.vi"("error in (no error)"=w455, "Enable Output (T: Enable)"=FALSE, "VISA resource name"=w457) -> ("error out"=w465:errorcluster, "VISA resource name out"=w464:refnum<visa-resource-name>)  [unwired: 7 in]
                n311 = call "Close.vi"("error in (no error)"=w465, "VISA resource name"=w464) -> ()  [unwired: 9 in, 1 out]
              }
            }
          }
          event "Step": Value Change {
            n312 = event-data() -> ()  [unwired: 1 in, 6 out]
            n313 = case shown="True" "Step" {
              frame False {
              }
              frame True {
                w529 = 1000 ("oversample (0)")
                w541 = u16 1 items=["Voltage", "Current"] ("Source Mode  (0: Voltage)")
                w546 = u16 1 items=["Voltage", "Current"] ("Source Mode  (0: Voltage)")
                w549 = u16 1 items=["Volts", "Current", "Resistance"] ("Function (0: Volts)")
                w552 = u16 0 items=["Volts", "Current", "Resistance"] ("Function (0: Volts)")
                n314 = local read "Detector Resource"() -> (w525:refnum<visa-resource-name>)
                n315 = property on="Oversample" class="DigNum (strict)"() -> (error out=w537:errorcluster, "Value"=w520:i32)  [unwired: 2 in, 1 out]
                n316 = call "Set OverSample.vi"("error in (no error)"=w537, "oversample (0)"=w529, "VISA resource name"=w525) -> ("error out"=w538:errorcluster)  [unwired: 7 in, 1 out]
                n317 = local read "CurrentSource"() -> (w545:refnum<visa-resource-name>)
                n318 = call "Initialize.vi"("error in (no error)"=w538, "ID Query (True)"=FALSE, "VISA resource name"=w545) -> ("error out"=w562:errorcluster, "VISA resource name out"=w561:refnum<visa-resource-name>)  [unwired: 7 in]
                n319 = call "Configure Measurement.vi"("error in (no error)"=w562, "Enable Auto Range (T:Enable)"=TRUE, "Function (0: Volts)"=w552, "VISA resource name"=w561) -> ("error out"=w556:errorcluster, "VISA resource name out"=w555:refnum<visa-resource-name>)  [unwired: 6 in]
                n320 = call "Configure Measurement.vi"("Manual Range (1.0)"=1e-07, "error in (no error)"=w556, "Enable Auto Range (T:Enable)"=FALSE, "Function (0: Volts)"=w549, "VISA resource name"=w555) -> ("error out"=w557:errorcluster, "VISA resource name out"=w558:refnum<visa-resource-name>)  [unwired: 5 in]
                n321 = call "Configure Output.vi"("Source Mode  (0: Voltage)"=w546, "error in (no error)"=w557, "Output Level (0)"="Current 1", "VISA resource name"=w558) -> ("error out"=w559:errorcluster, "VISA resource name out"=w560:refnum<visa-resource-name>)  [unwired: 6 in]
                n322 = call "Enable Output.vi"("error in (no error)"=w559, "Enable Output (T: Enable)"=TRUE, "VISA resource name"=w560) -> ("error out"=w544:errorcluster, "VISA resource name out"=w540:refnum<visa-resource-name>)  [unwired: 7 in]
                n323 = call <userlib>:"Wait (ms)__ogtk.vi"("error in (no error)"=w544, "milliseconds to wait"="Delay 1 (ms)") -> ("error out"=w542:errorcluster)  [unwired: 8 in, 1 out]
                n324 = call "Configure Output.vi"("Source Mode  (0: Voltage)"=w541, "error in (no error)"=w542, "Output Level (0)"="Current 2", "VISA resource name"=w540) -> ("error out"=w536:errorcluster, "VISA resource name out"=w522:refnum<visa-resource-name>)  [unwired: 6 in]
                n325 = call "Get BURST.vi"("error in (no error)"=w536, "chan (0)"="chan (0)", "VISA resource name"=w525) -> ("error out"=w534:errorcluster, "subarray"=w527:dbl[], "VISA resource name out"=w533:refnum<visa-resource-name>)  [unwired: 5 in, 1 out]
                n326 = for {
                  tunnel: w527 -> [_] mode=indexing
                  tunnel: [w563] -> w532 mode=indexing
                  i -> [w563]
                }
                n327 = call "Get Time.vi"("error in (no error)"=w534, "VISA resource name"=w533) -> ("error out"=w523:errorcluster, "output"=w531:i32, "VISA resource name out"=w519:refnum<visa-resource-name>)  [unwired: 7 in]
                n328 = Divide(x=w531, y=w529) -> (x/y=w530:dbl)
                n329 = Multiply(x=w530, y=w532) -> (x*y=w528:dbl[])
                n330 = Bundle(w528, "subarray"=w527) -> (→"Step Response":cluster{dbl[], "subarray":dbl[]})  [unwired: 1 in]
                n331 = call "Enable Output.vi"("error in (no error)"=w523, "Enable Output (T: Enable)"=TRUE, "VISA resource name"=w522) -> ("error out"=w521:errorcluster)  [unwired: 7 in, 1 out]
                n332 = call "Set OverSample.vi"("error in (no error)"=w521, "oversample (0)"=w520, "VISA resource name"=w519) -> ()  [unwired: 7 in, 2 out]
              }
            }
          }
          event "Exit": Value Change {
            # "If stage is connected, go to reference position and then exit"
            n333 = event-data() -> ()  [unwired: 1 in, 6 out]
            n334 = flat-sequence {
              frame #0 {
                n335 = local write "Measurement Mode"(T2."Stage Drive" ("Measurement Mode")) -> ()
              }
              frame #1 {
                n336 = local read "connected"() -> (w565:bool)
                n337 = case shown="True" w565 {
                  frame False {
                  }
                  frame True {
                    n338 = local read "MCSChannel"() -> (w567:i8)
                    n339 = local read "Handle"() -> (w566:refnum<class "SA_CTL.lvclass">)
                    n340 = call "SA_CTL_Move.vi"("moveValue"=i64 0, "SA_CTL_Handle"=w566, "channel"=w567) -> ("error out"=w568:errorcluster)  [unwired: 12 in]
                    n341 = while {
                      tunnel: w568 -> [w577]
                      tunnel: w567 -> [w576]
                      tunnel: w566 -> [w575]
                      tunnel: [w571] -> _
                      stop <- w573 stop-if-true
                      n342 = call "SA_CTL_GetChannelState.vi"("SA_CTL_Handle"=w575, "channel"=w576, "error in (no error)"=w577) -> ("ChannelState"=w574:i32, "error out"=w571:errorcluster)  [unwired: 11 in]
                      n343 = And(x=1, y=w574) -> (x .and. y?=w570:i32)
                      n344 = Equal To 0?(x=w570) -> (x = 0?=w573:bool)
                    }
                  }
                }
              }
              frame #2 {
                n345 = local write "exit"(TRUE) -> ()
              }
            }
          }
          event Panel Close? {
            # "Discard \"Panel Close?\" event\n\nto leave program through\n graceful route"
            # "NOTE:\nMake sure not to use the red \"Abort Execution\" button in the\nLabVIEW menu to abort the application execution.\nDoing so will not close the device connection with the consequence that\na re-open after the next application start will fail."
            # "\"Panel Close\" (\"X\") was clicked by the user:\nWe discard the close command and set an \"exit\" flag. This gives us the change to proper disconnect the device and clean up the application before closing the window."
            # "Trap \"Panel Close\" instruction and exit program gracefully"
            n346 = event-data() -> ()  [unwired: 1 in, 4 out]
            n347 = local write "exit"(TRUE ("exit")) -> ()
            n348 = event-data("Discard?"=TRUE) -> ()  [unwired: 1 in, 1 out]
          }
        }
        n349 = local read "exit"() -> (w59:bool)
      }
      n350 = disable-structure shown="Disabled" {
        frame Disabled {
          n351 = node-c288("Delay(mS)") -> (w28:T4)  [unwired: 9 in]
          n352 = timed-loop {
            shift-right: [w31] -> _
            shift-left: _ -> [w30]
            timing: w28 -> [_]
            timing-out: [_] -> w27
            stop <- w33 stop-if-true
            # "positioner information loop"
            n353 = node-c288() -> ()  [unwired: 1 in, 1 out]
            n354 = local read "connected"() -> (w32:bool)
            n355 = case shown="True" w32 {
              frame False {
              }
              frame True {
                # "note: clear specific error code is only available since LV2014\nthus we do this manually"
                # "Individual errors can be ignored with the \"Clear Error\"\nfunction if they are not of interest."
                # "All VIs may be used parallel from different threads (\"while loops\")\nThe DLL handles the correct serializing."
                # "position polling: Reading the position requires a sensor to be present and enabled (or in powersave mode)."
                n356 = local read "MCSChannel"() -> (w45:i8)
                n357 = local read "Handle"() -> (w46:refnum<class "SA_CTL.lvclass">)
                n358 = call "SA_CTL_GetPosition.vi"("SA_CTL_Handle"=w46, "channel"=w45) -> ("Position"=w44:i64, "error out"=w48:errorcluster)  [unwired: 12 in]
                n359 = Divide(x=w44, y=i64 1000000 ("x")) -> (x/y=→"Position (µm)":dbl)
                n360 = Multiply(x=1e-06, y=w44) -> (x*y=w43:dbl)
                n361 = case shown="True" "Enable" {
                  tunnel: w43 -> [_ w51]
                  frame False {
                  }
                  frame True {
                    "Waveform Chart" <- w51
                  }
                }
                n362 = call "SA_CTL_GetChannelState.vi"("SA_CTL_Handle"=w46, "channel"=w45, "error in (no error)"=w48) -> ("ChannelState"=w41:i32, "error out"=w47:errorcluster)  [unwired: 11 in]
                "ChannelState" <- w41
                n363 = Number To Boolean Array(number=w41) -> (Boolean array=w40:bool[])
                n364 = Array To Cluster(array=w40) -> (cluster=→"PositionerStatus":T8)
                n365 = Unbundle By Name(w47) -> ("code"=w49:i32)
                n366 = case shown="103, 104" w49 {
                  tunnel: w47 -> [w52 w54]
                  tunnel: [w52 w53] -> w50
                  frame Default {
                  }
                  frame 259, 260 {
                    # "SA_CTL_ERROR_NO_SENSOR_PRESENT\nSA_CTL_ERROR_SENSOR_DISABLED"
                    n367 = call <vilib>:"Clear Errors.vi"("error in (no error)"=w54) -> ("error out"=w53:errorcluster)  [unwired: 5 in, 1 out]
                  }
                }
                n368 = local write "Error Out"(w50) -> ()
              }
            }
            n369 = Tick Count (ms)() -> (millisecond timer value=w31:u32)
            n370 = local read "exit"() -> (w33:bool)
            n371 = Subtract(x=w31, y=w30) -> (x-y=→"Elapsed (ms)":u32)
            n372 = node-c288() -> ()  [unwired: 1 in, 1 out]
          }
          n373 = node-c288(w27) -> ()  [unwired: 1 out]
        }
        frame Enabled {
        }
      }
    }
    frame #2 {
      # "Cleanup and Shutdown"
      n374 = local read "connected"() -> (w581:bool)
      n375 = case shown="True" w581 {
        frame False {
        }
        frame True {
          # "Also power off and close detector SCPI EGSE"
          # "always make sure to close the connection\nto the device before quitting the program"
          n376 = local read "Detector Resource"() -> (w586:refnum<visa-resource-name>)
          n377 = call "Set Power.vi"("Power (0)"=FALSE, "VISA resource name"=w586) -> ("error out"=w583:errorcluster, "VISA resource name out"=w587:refnum<visa-resource-name>)  [unwired: 8 in]
          n378 = property on="Power" class="Bool (strict)"(error in=w583, "Value"=FALSE ("Power")) -> (error out=w584:errorcluster)  [unwired: 1 in, 1 out]
          n379 = local read "Handle"() -> (w588:refnum<class "SA_CTL.lvclass">)
          n380 = call "Close.vi"("error in (no error)"=w584, "VISA resource name"=w587) -> ()  [unwired: 9 in, 1 out]
          n381 = call "SA_CTL_Close.vi"("SA_CTL_Handle"=w588) -> ()  [unwired: 10 in, 1 out]
        }
      }
    }
  }
